vi "Pick&Place_ladder_shih_v3.vi"() -> ()   [LabVIEW 2016]
uses:
  Classes/Controllers/I-O/Copy of NI-DAQ Folder/NI-DAQ.lvclass
  D:/INTT/V1/Classes/Controllers/I-O/Copy of I-O Folder/I-O.lvclass
  Classes/Controllers/Dispenser/Copy of Ultimus V2 Folder/Ultimus V2.lvclass
  <vilib>/Analysis/coordinate.llb/2D Cartesian Coordinate Rotation (Scalar).vi
  <vilib>/Utility/file.llb/Read Delimited Spreadsheet (DBL).vi
  <vilib>/Utility/file.llb/Write Delimited Spreadsheet (DBL).vi
  Classes/Controllers/Motion/Copy of Motion Folder/Motion.lvclass
  Classes/Controllers/Camera/Copy of Controller Folder/Controller.lvclass
  <vilib>/Analysis/NI_AALPro.lvlib
  Classes/Controllers/I-O/Copy of I-O Folder/I-O.lvclass
panel:
  out "FROM Detail !!! Center of module on stave 2":dbl[](array[numeric])
  out "FROM Detail !! measured stave size":dbl[](array[numeric])
  in  "Align Stave in detail":bool
  in  "check height?":bool
  in  "Uttimus presssure":i64=10
  out "Status":bool
  out "measured HDI top-left position":dbl[][](array[numeric])
  in  "HDI vacuum channel":i32=18
  in  "vacuum":bool=TRUE
  in  "HDI vacuum":bool
  out "measured stave size":dbl[](array[numeric])
  out "Stave mark":dbl[][](array[numeric])
  out "Center of module on stave":dbl[](array[numeric])
  out "Center of HDI from alignment mark":dbl[](array[numeric])
  out "Measured HDI size":dbl[][](array[numeric])
  out "module position on stave":dbl[][](array[numeric])
  in  "Default Stave dimension":dbl[](array[numeric])=[34.0, 472.0, -0.335295, -0.000320234]
  in  "Default Stave upper left mark":dbl[](array[numeric])=[584.376, 675.576, 70.9882, 0.000840064]
  out "Needle parking position":dbl[](array[numeric])
  in  "Uppler / Lower Stave":bool=TRUE
  out "Gantry current position":dbl[](array[numeric])
  in  "READ Position":bool
  in  "Needle Height Compenstation\n(glue gap)":dbl=0.33
  in  "Needle Alignment":bool
  in  "Parking position":dbl[](array[numeric])=[625.0, 625.0, 0.0, 0.01]
  in  "GOTO":bool
  in  "Default Pickup Tool Position":dbl[][](array[numeric])=[[152.226, 682.729, 36.8129, -0.0151898], [700.0, 800.0, 20.0, 0.01]]
  in  "Number of module \nto be assembled":i32=1
  in  "Default HDI alignment \nmark position":dbl[](array[numeric])=[448.322, 976.582, 74.9872, 0.000191129]
  in  "Default HDI size":dbl[](array[numeric])=[24.2437, 231.446, -0.099339, 0.000191129]
  out "# of tasks excuted":i32
  out "module on tray position":dbl[][](array[numeric])
  out "PickupTool \nCenterPosition":dbl[](array[numeric])
  in  "Inititalize":bool
  in  "Pick and place":bool
  in  "Deposit Glue":bool
  in  "Measure Pickup Tools":bool
  in  "Align Stave":bool
  out "default module position on stave":dbl[][](array[numeric])
  in  "Stop":bool
  in  "Measure HDI":bool
  # "Ladder Assembly"
  # "Lower\nmodule"
  # "Upper\nmodule"
  # "Sensor 0.32 -> 200 micron glue thickness\nChips 0.37-> 140 micron glue thickness"
  # "ACTIONS"
  # "Stave infomation"
  # "Module infomation"
  # "Pick and Place"
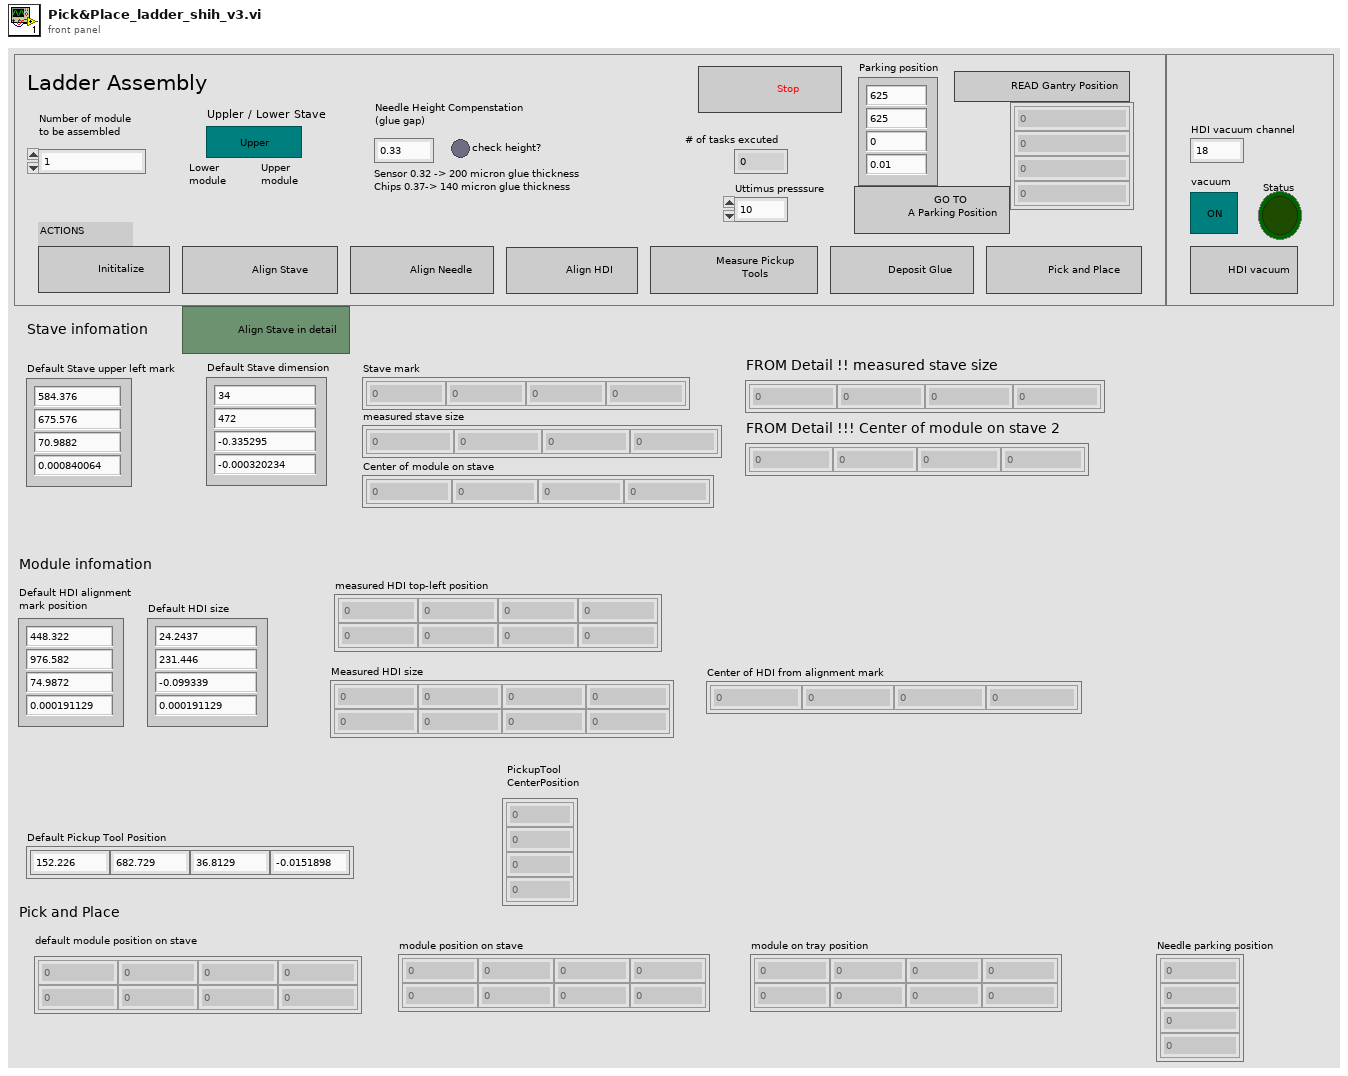
[diagram p1: front panel]
types:
  T1 = typedef "Controller.lvclass/Controllers.ctl" = cluster{"Copy of Motion.lvclass":refnum<class "Motion.lvclass">, "Copy of I-O.lvclass":refnum<class "I-O.lvclass">, "Copy of Dispenser.lvclass":refnum<class "Dispenser.lvclass">}
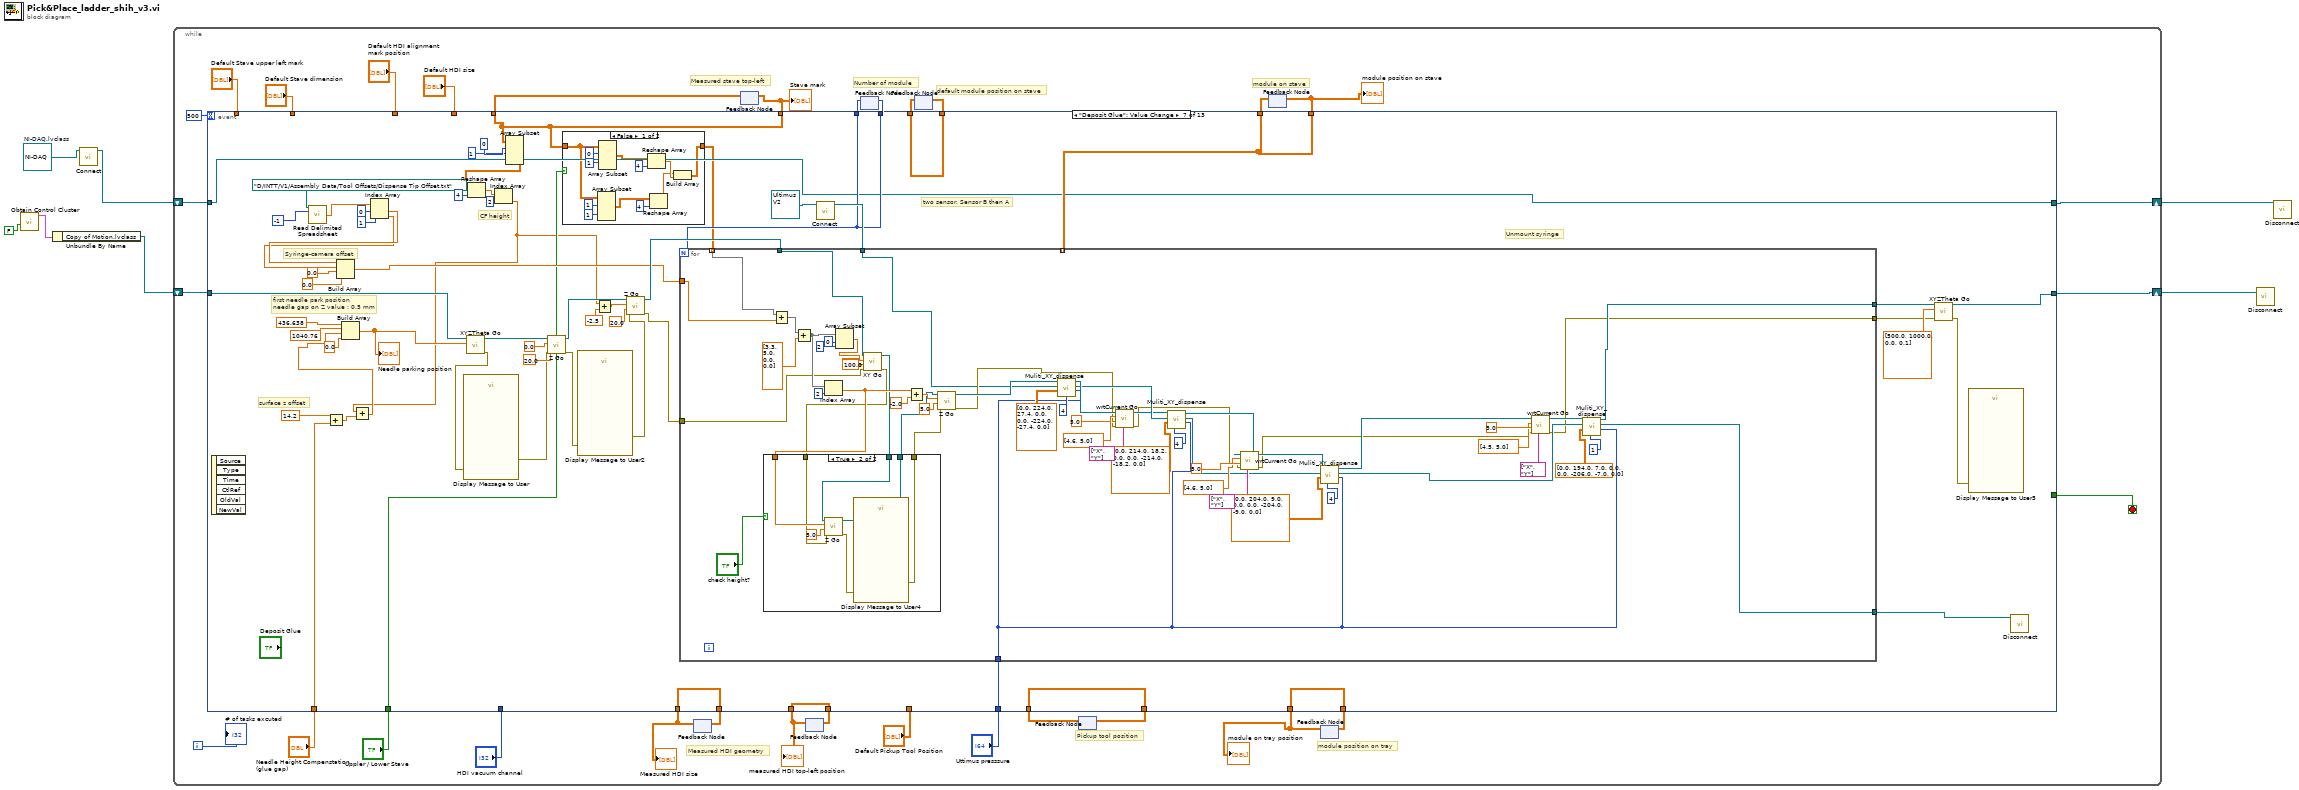
[diagram p0: block diagram]
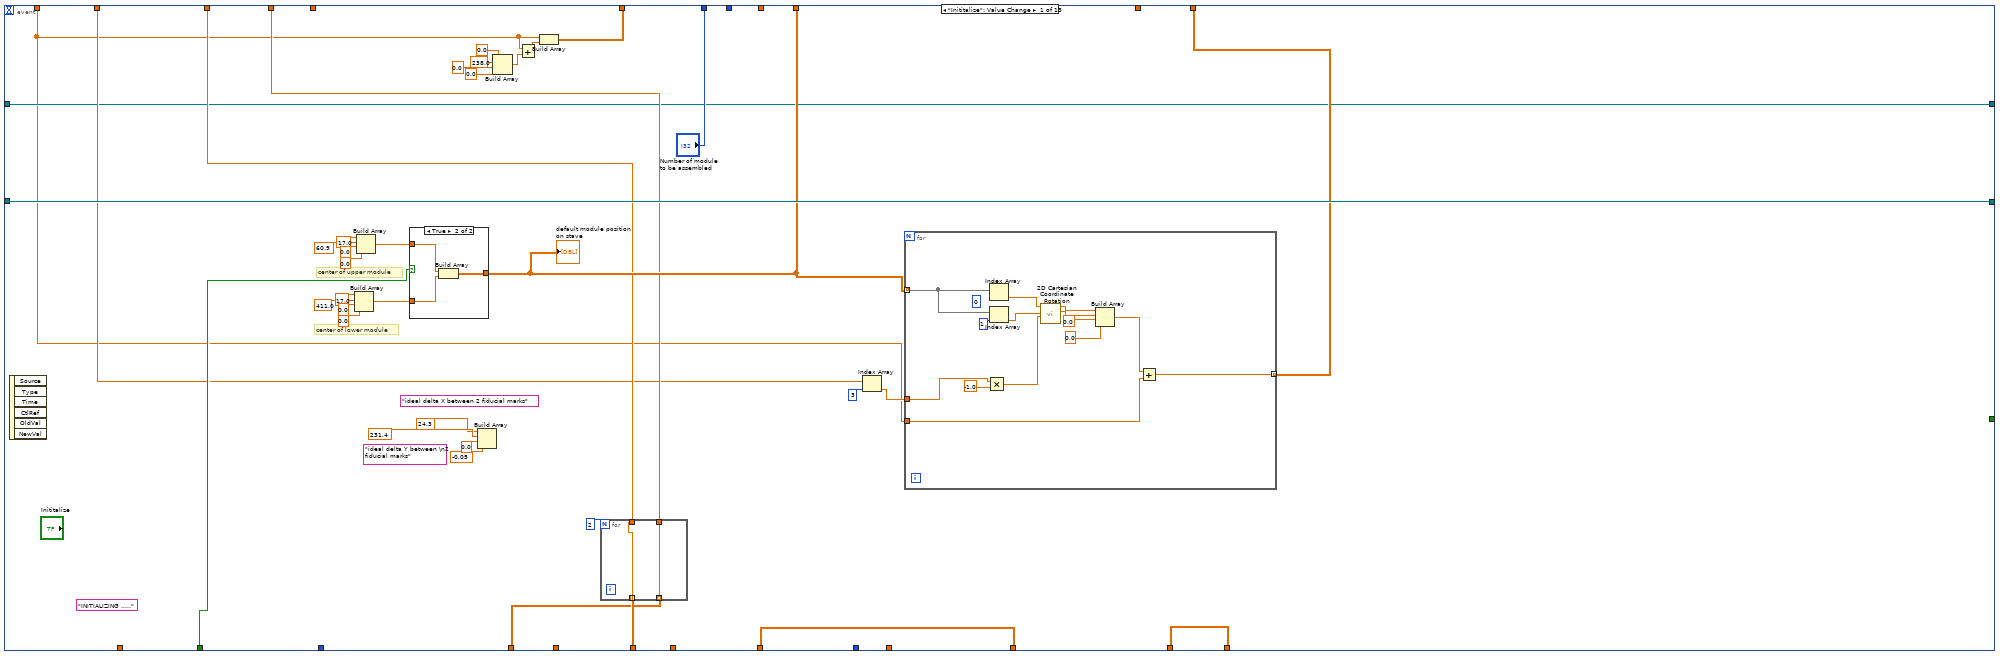
[diagram p2: hidden frame]
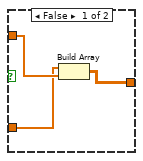
[diagram p3: hidden frame]
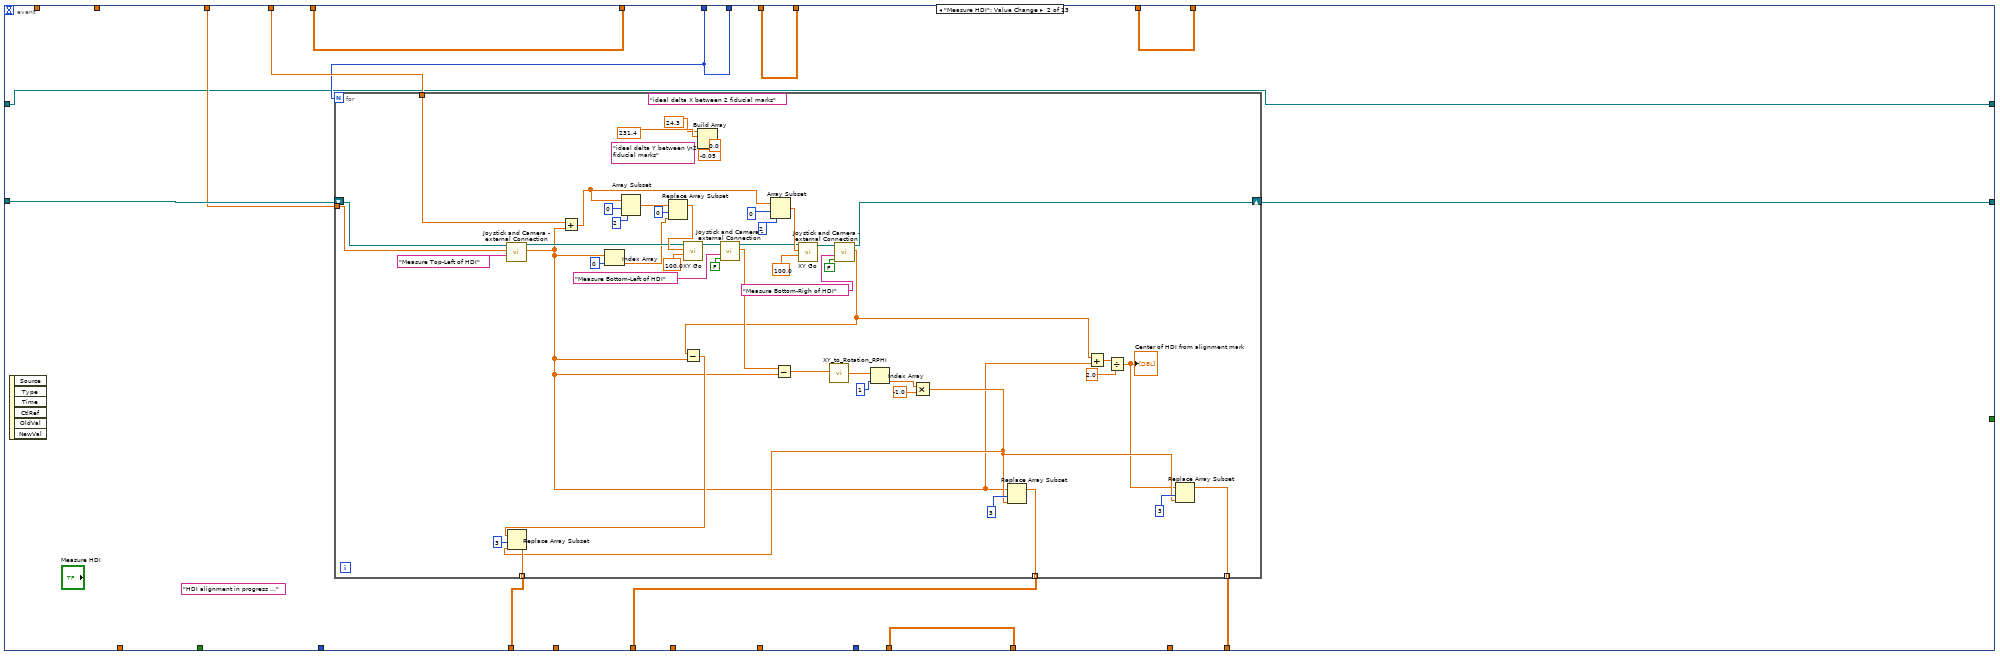
[diagram p4: hidden frame]
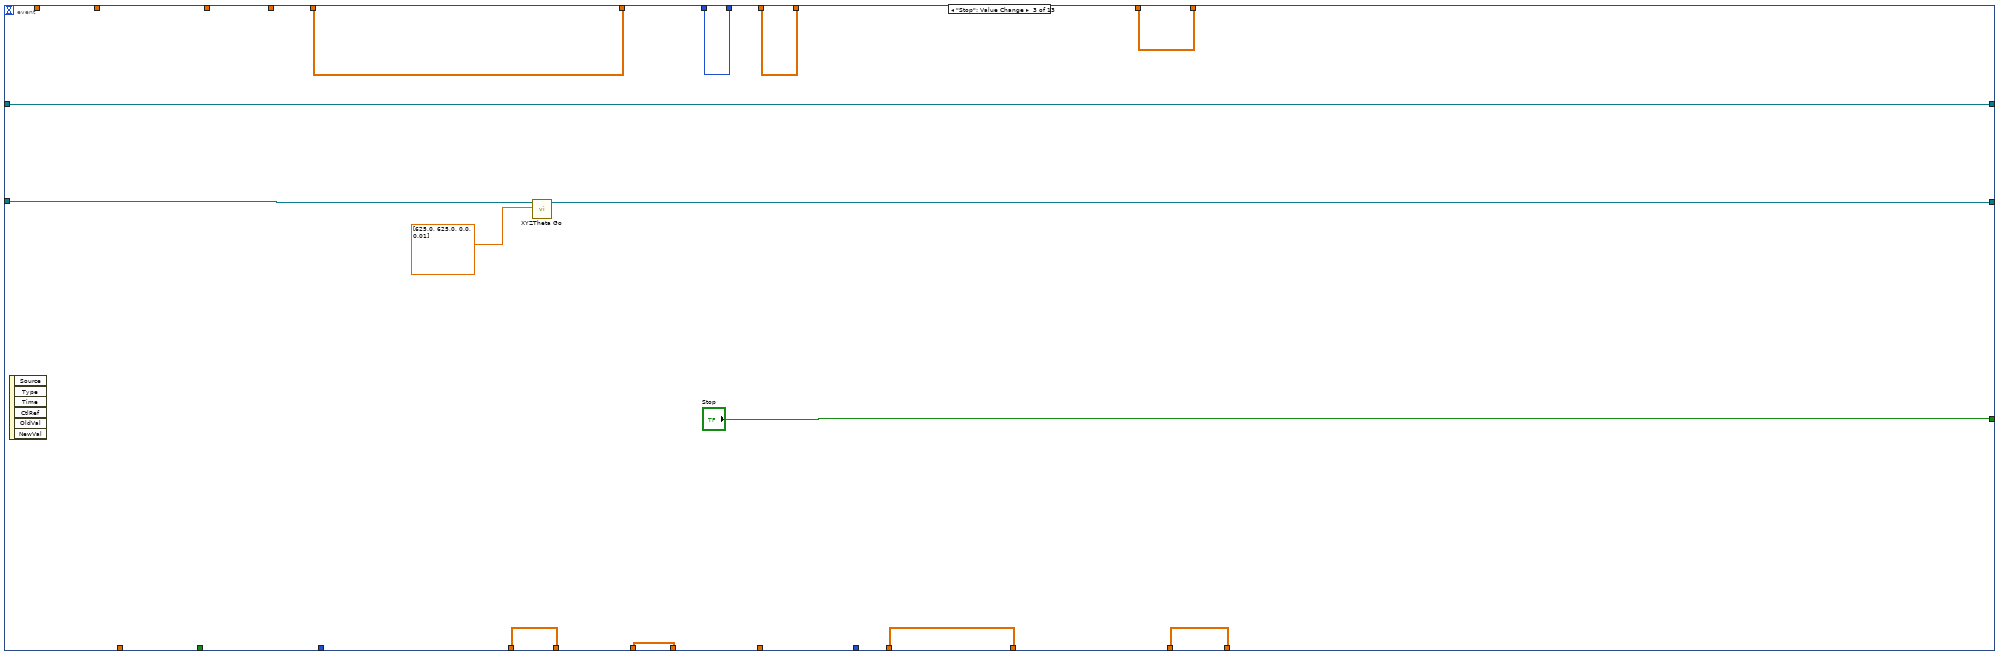
[diagram p5: hidden frame]
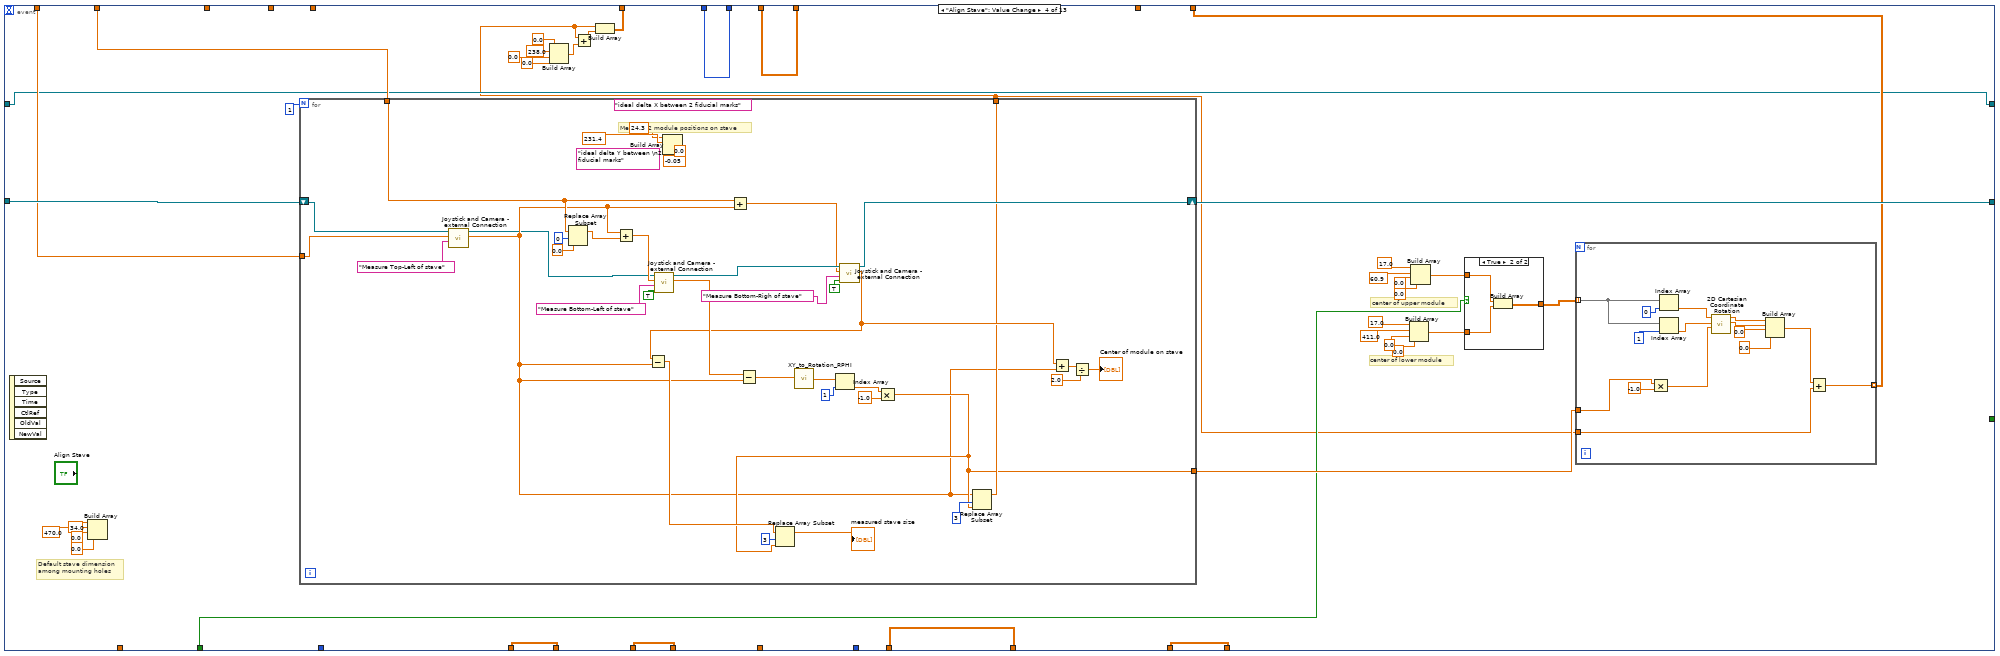
[diagram p6: hidden frame]
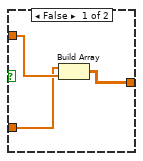
[diagram p7: hidden frame]
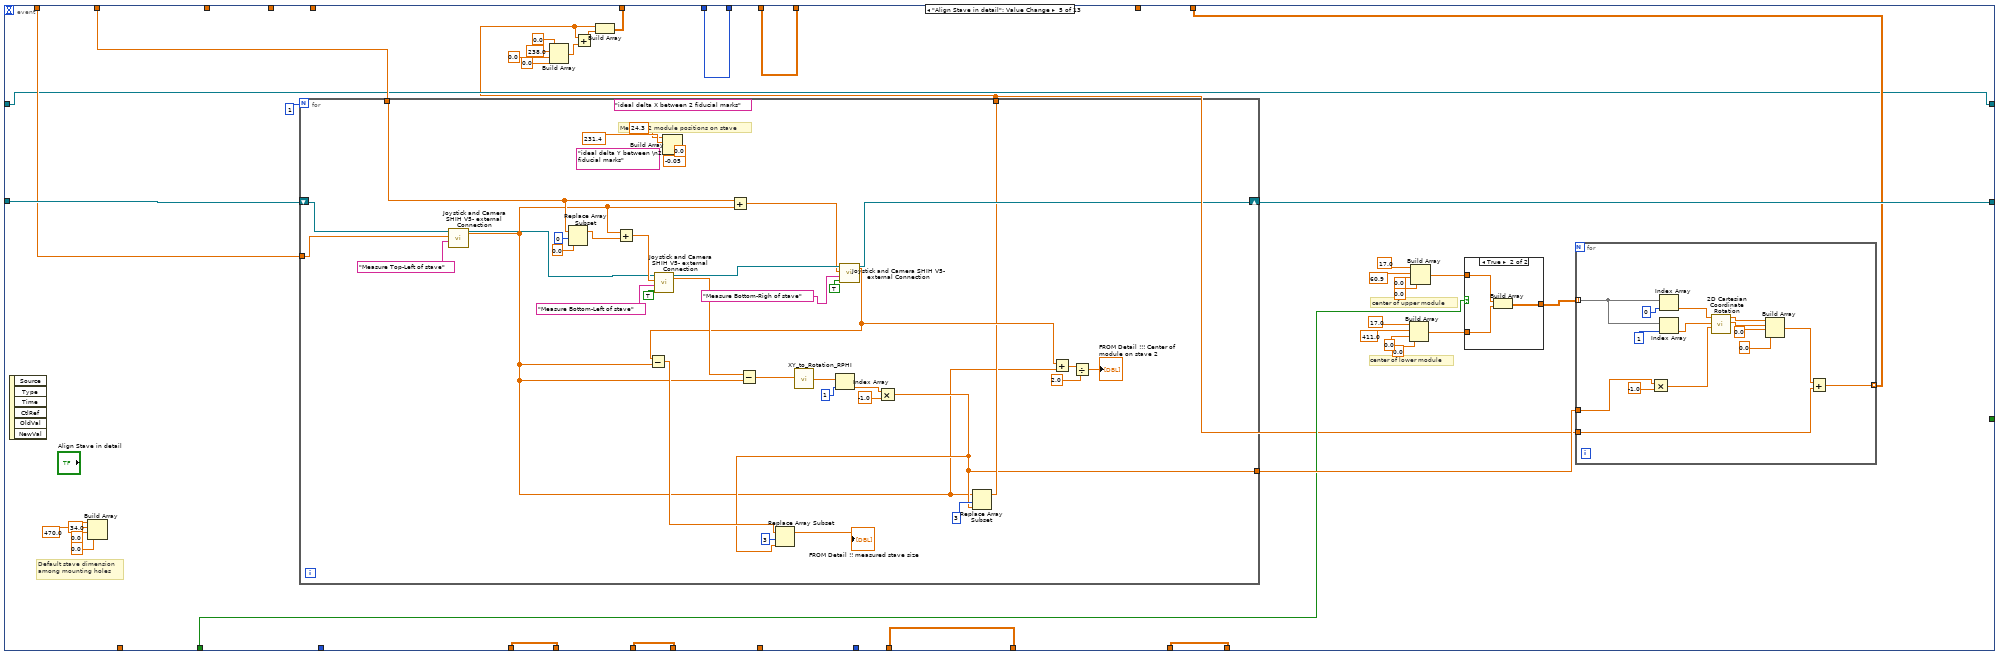
[diagram p8: hidden frame]
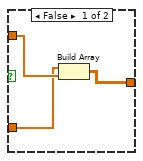
[diagram p9: hidden frame]
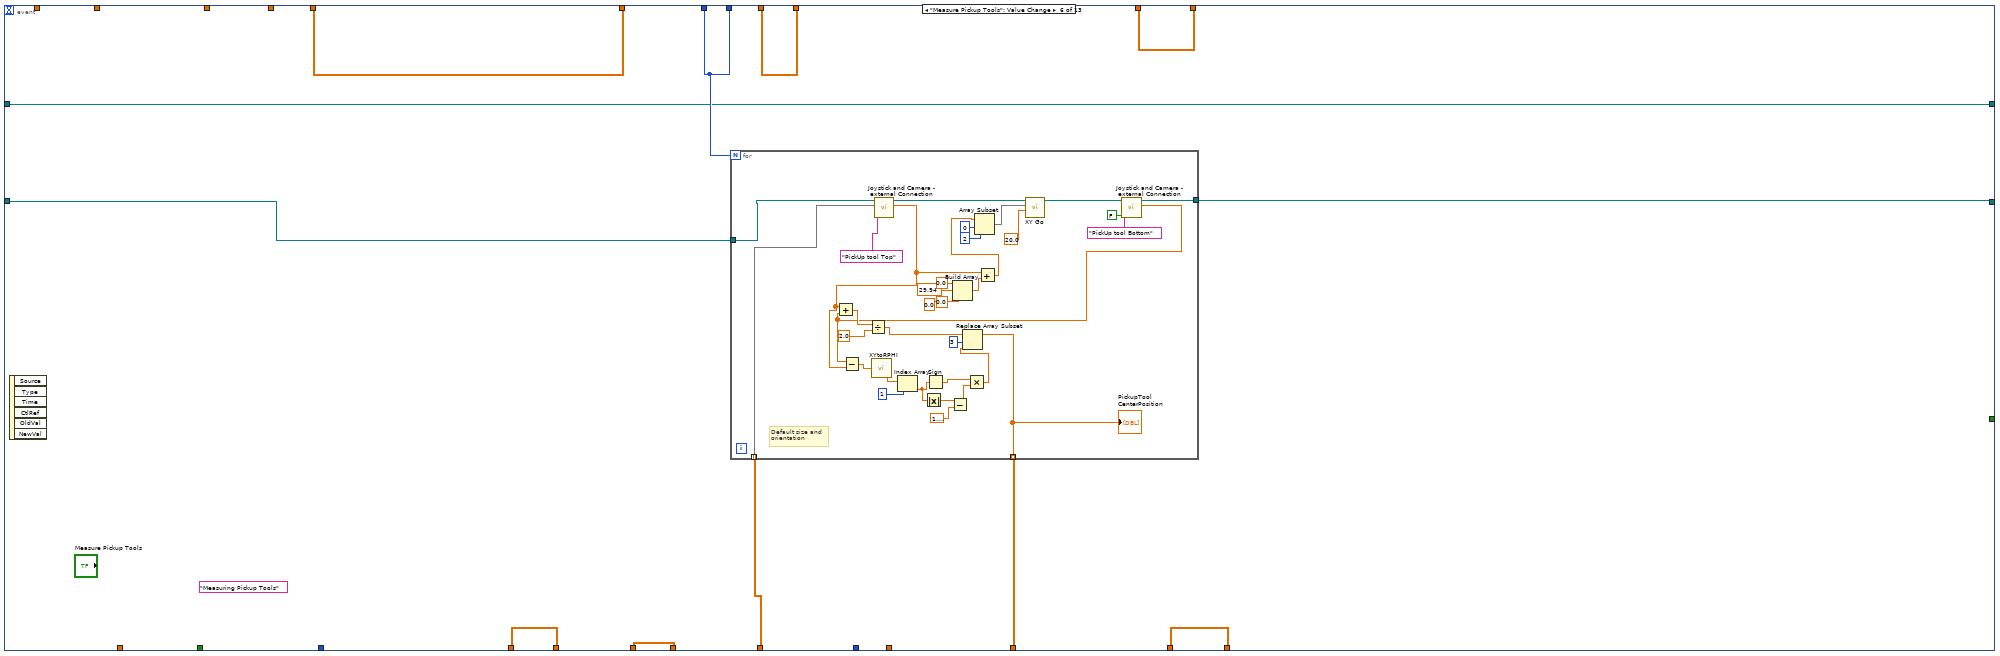
[diagram p10: hidden frame]
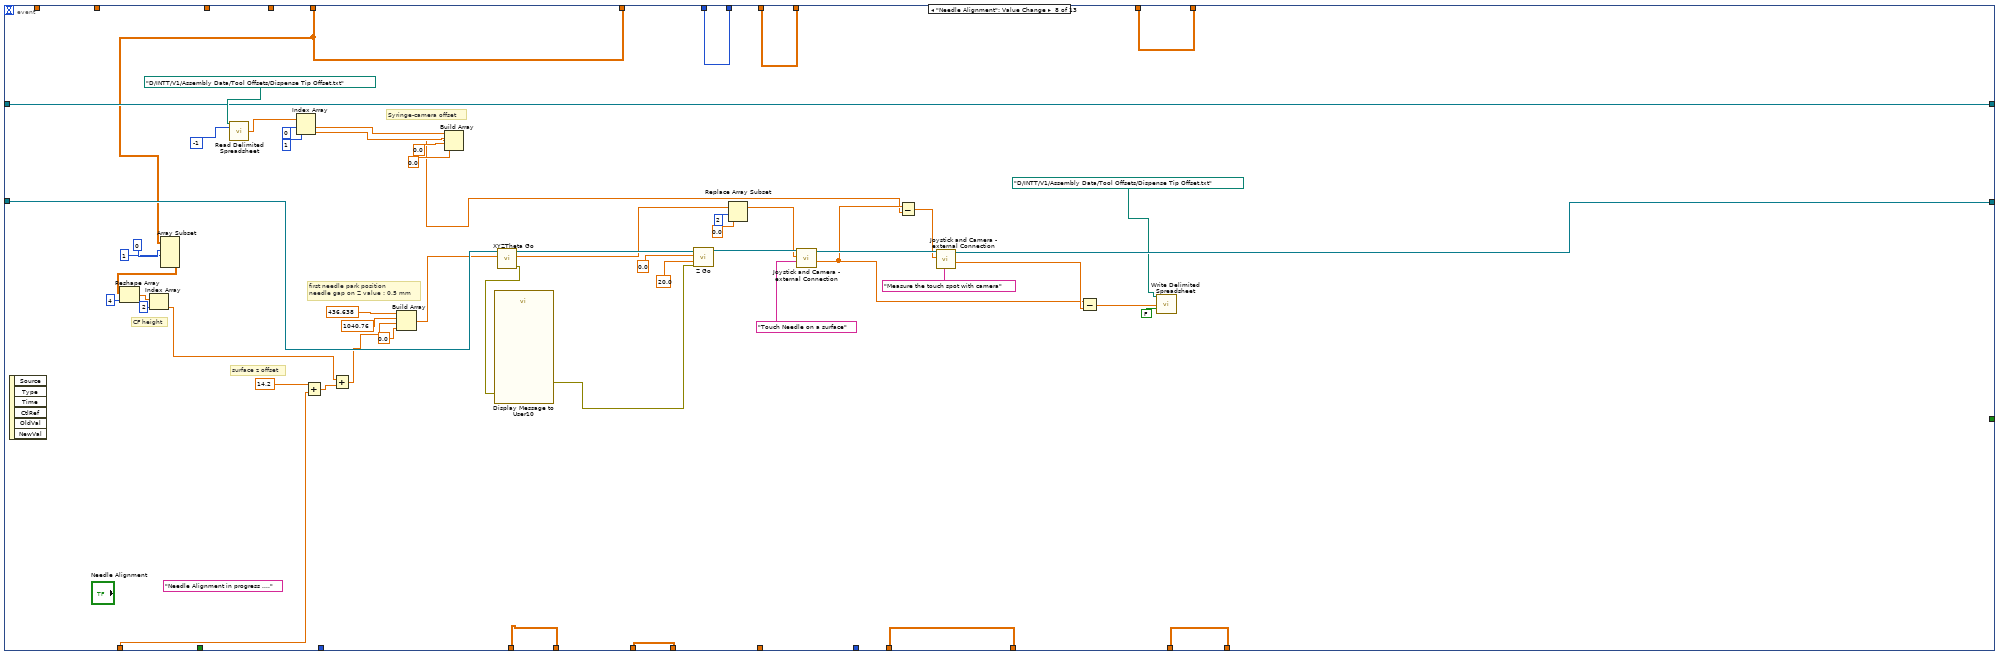
[diagram p13: hidden frame]
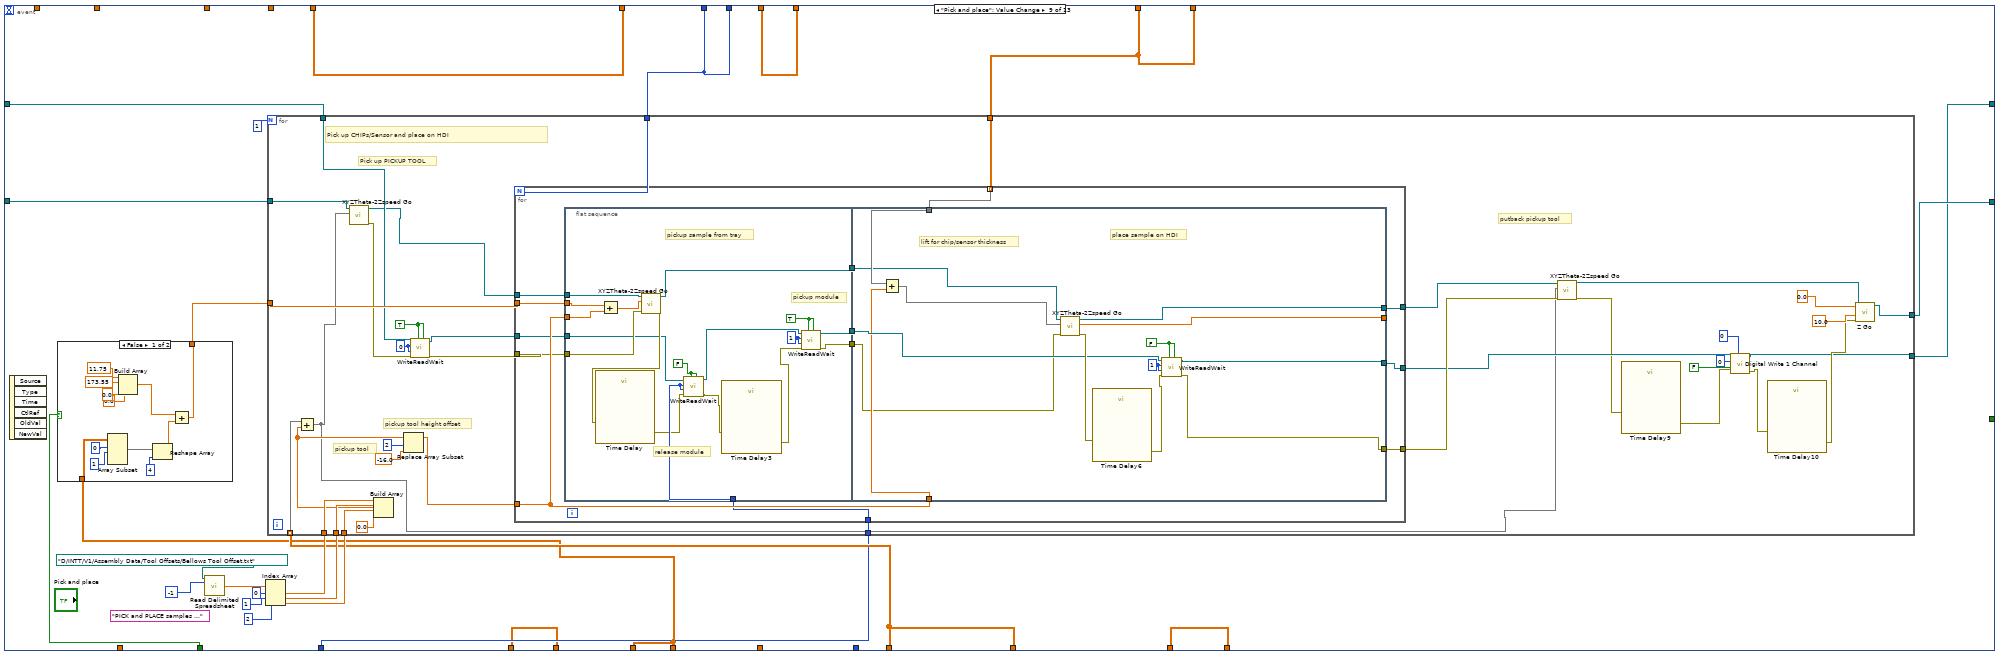
[diagram p14: hidden frame]
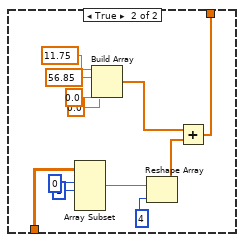
[diagram p15: hidden frame]
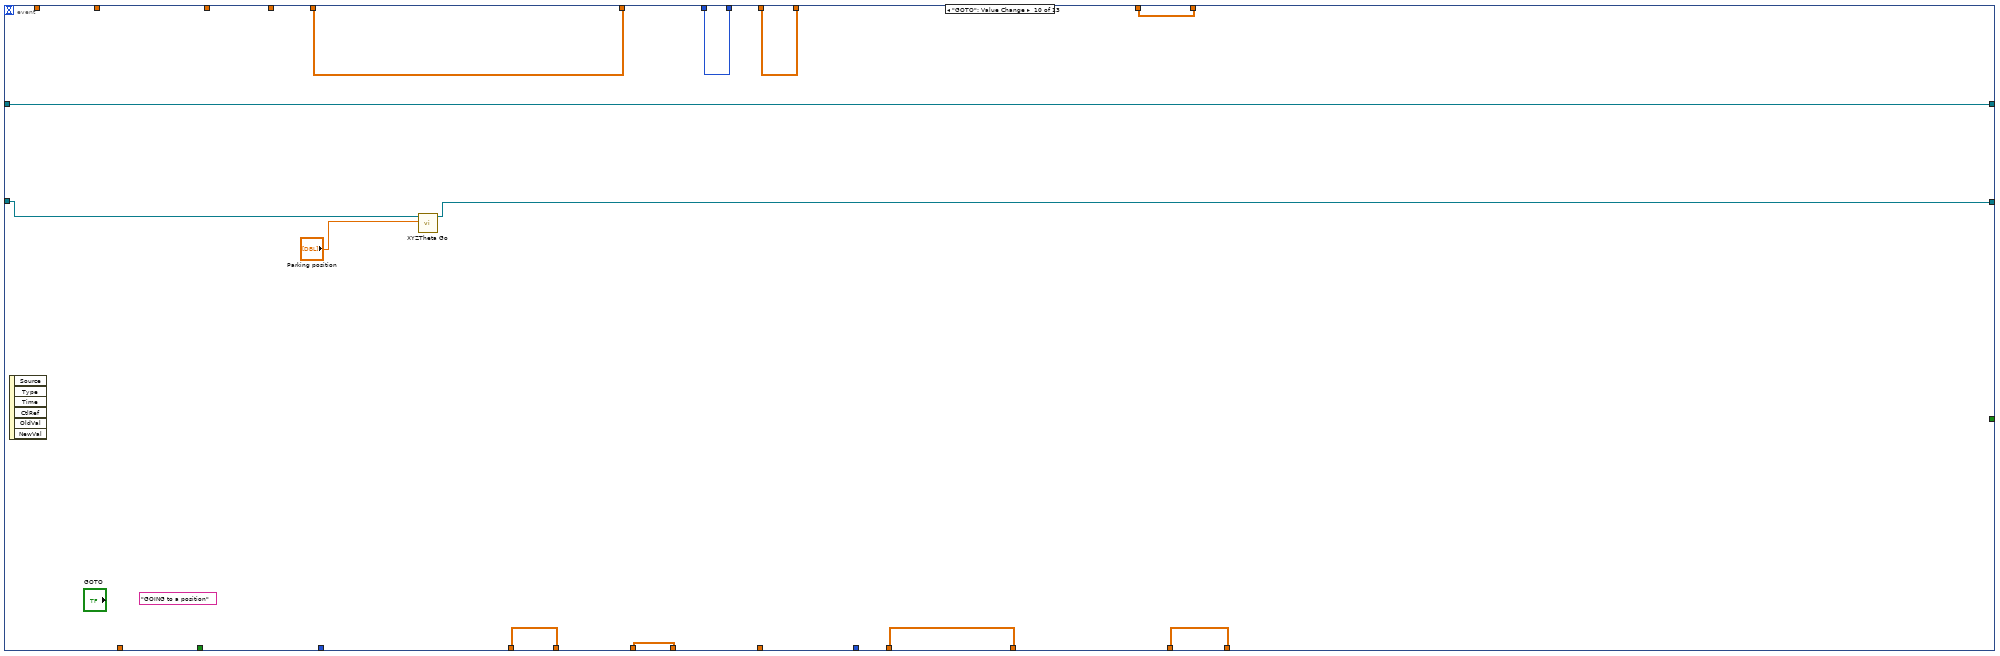
[diagram p16: hidden frame]
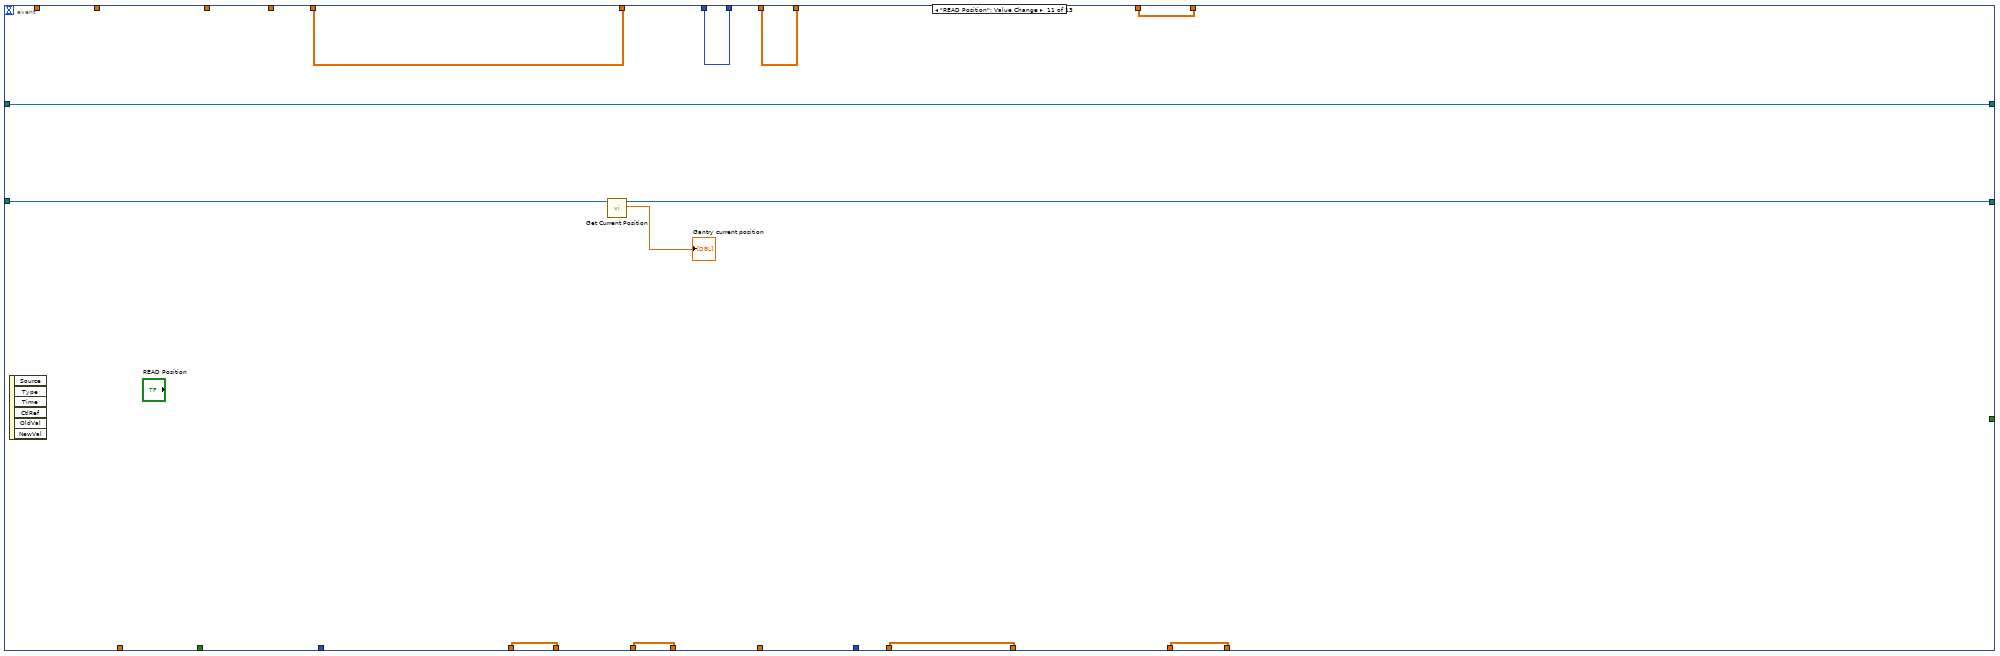
[diagram p17: hidden frame]
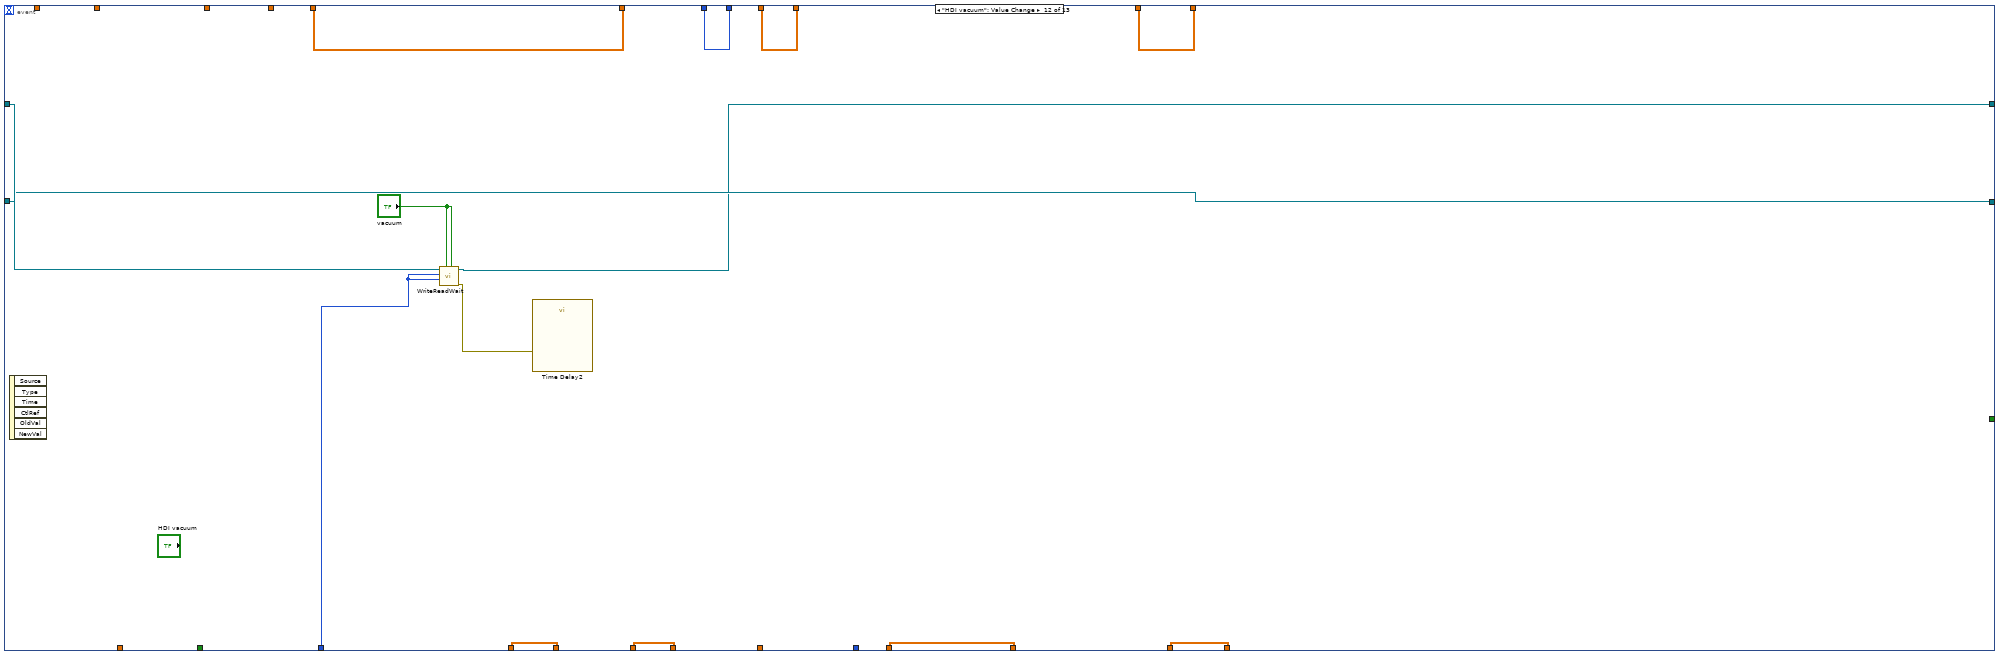
[diagram p18: hidden frame]
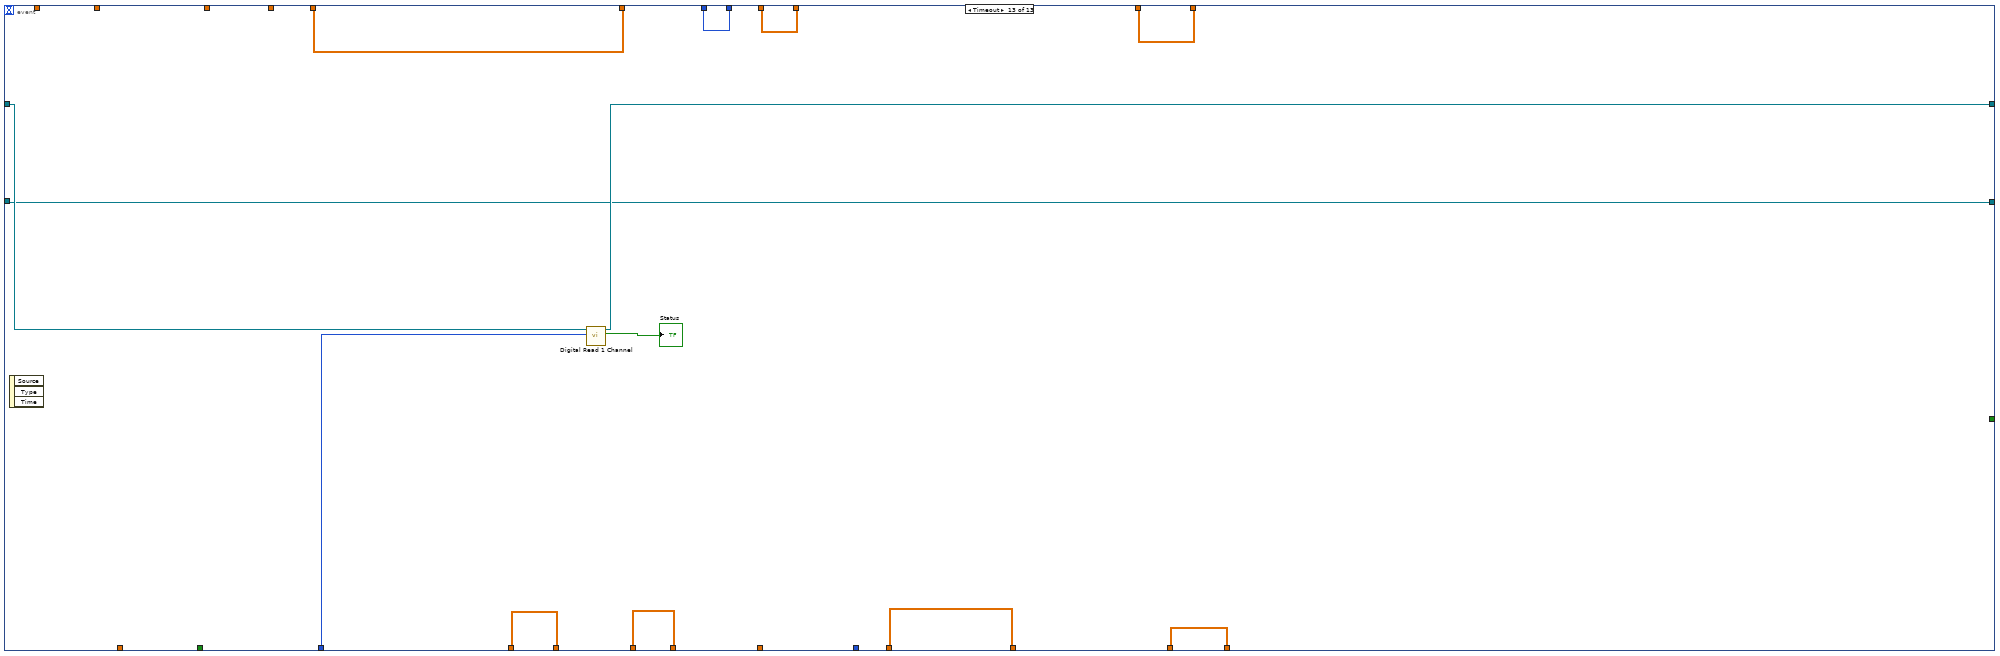
[diagram p19: hidden frame]
diagram:
  w3 = refnum<class "NI-DAQ.lvclass"> refnum  # NI-DAQ.lvclass
  n1 = call "Obtain Control Cluster.vi"("I/O"=FALSE) -> ("Control Out"=w7:T1)  [unwired: 10 in]
  n2 = Unbundle By Name(w7) -> ("Copy of Motion.lvclass"=w5:refnum<class "Motion.lvclass">)
  n3 = call-dynamic "Connect.vi"("NI-DAQ in"=w3) -> ("NI-DAQ out"=w2:refnum<class "NI-DAQ.lvclass">)  [unwired: 9 in, 1 out]
  n4 = while {
    shift-right: [w32] -> w4
    shift-left: w5 -> [w39]
    shift-right: [w11] -> w1
    shift-left: w2 -> [w15]
    i -> [w31]
    stop <- w38 stop-if-true
    # "default module position on stave"
    # "Pickup tool position"
    # "Number of module"
    # "Measured HDI geometry"
    # "module position on tray"
    # "Measured stave top-left"
    # "module on stave"
    n5 = feedback #1() -> (w36:dbl[][])  [unwired: 1 in]
    n6 = feedback #2() -> (w37:dbl[][])  [unwired: 1 in]
    n7 = feedback #3() -> (w12:dbl[][])  [unwired: 1 in]
    n8 = feedback #4() -> (w30:i32)  [unwired: 1 in]
    n9 = feedback #5() -> (w25:dbl[][])  [unwired: 1 in]
    n10 = feedback #6() -> (w33:dbl[][])  [unwired: 1 in]
    n11 = feedback #7() -> (w19:dbl[][])  [unwired: 1 in]
    n12 = feedback #8() -> (w23:dbl[][])  [unwired: 1 in]
    "module on tray position" <- w23
    n13 = event shown="[6] \"Deposit Glue\": Value Change" {
      selector: _ -> [_ _ _ _ _ _ _ _ _ _ _ _ _]
      dyn-events: _ -> [_ _ _ _ _ _ _ _ _ _ _ _ _]
      timeout: 500 -> [_ _ _ _ _ _ _ _ _ _ _ _ _]
      tunnel: w39 -> [w73 w112 w174 w204 w300 w378 w451 w585 w629 w741 w759 w761 w782]
      tunnel: [_ _ "Stop" _ _ _ _ _ _ _ _ _ _] -> w38
      tunnel: [w40 w106 w169 w175 w271 w373 w413 w551 w607 w747 w755 w769 w781] -> w16
      tunnel: w37 -> [_ w106 w169 _ _ w373 w413 w551 w607 w747 w755 w769 w781]
      tunnel: [w50 w104 w168 w200 w296 w372 w437 w588 w610 w744 w754 w763 w779] -> w17
      tunnel: w36 -> [_ _ w168 w200 w296 w372 w437 w588 w610 w744 w754 w763 w779]
      tunnel: w30 -> [_ w102 w171 w205 w301 w369 w440 w590 w614 w746 w756 w767 w774]
      tunnel: [w55 w103 w166 w207 w303 w371 w439 w586 w617 w742 w752 w765 w776] -> w35
      tunnel: w23 -> [w55 _ w166 w207 w303 w371 w439 w586 w617 w742 w752 w765 w776]
      tunnel: [w71 w107 w167 w212 w308 w377 w438 w587 w618 w743 w753 w764 w777] -> w34
      tunnel: w33 -> [_ w107 w167 w212 w308 _ w438 w587 w618 w743 w753 w764 w777]
      tunnel: [w73 w111 w172 w201 w297 w376 w441 w577 w619 w739 w758 w761 w782] -> w32
      tunnel: ["Number of module \nto be assembled" w102 w171 w205 w301 w369 w440 w590 w614 w746 w756 w767 w774] -> w29
      tunnel: "Default HDI alignment \nmark position" -> [w53 w110 _ _ _ _ _ _ _ _ _ _ _]
      tunnel: "Default HDI size" -> [w52 w109 _ _ _ _ _ _ _ _ _ _ _]
      tunnel: [w60 w108 w170 w206 w302 w374 w436 w589 w616 w745 w757 w768 w780] -> w26
      tunnel: w25 -> [_ w108 w170 w206 w302 w374 w436 w589 w616 w745 w757 w768 w780]
      tunnel: "Default Pickup Tool Position" -> [w71 _ _ _ _ w375 _ _ _ _ _ _ _]
      tunnel: "Uppler / Lower Stave" -> [w56 _ _ w185 w281 _ w421 _ w605 _ _ _ _]
      tunnel: "Default Stave upper left mark" -> [w41 _ _ w203 w299 _ _ _ _ _ _ _ _]
      tunnel: "Default Stave dimension" -> [w49 _ _ w202 w298 _ _ _ _ _ _ _ _]
      tunnel: [w57 w105 w164 w184 w280 w370 w435 w568 w606 w737 w749 w766 w775] -> w18
      tunnel: w19 -> [_ w105 w164 _ _ w370 w435 w568 w606 w737 w749 w766 w775]
      tunnel: w15 -> [w48 w100 w162 w183 w279 w367 w430 w566 w613 w736 w748 w773 w785]
      tunnel: [w48 w100 w162 w183 w279 w367 w430 w566 w612 w736 w748 w760 w783] -> w11
      tunnel: "HDI vacuum channel" -> [_ _ _ _ _ _ _ _ w611 _ _ w770 w784]
      tunnel: [w51 w101 w163 w199 w295 w368 w431 w567 w609 w738 w750 w762 w778] -> w13
      tunnel: w12 -> [_ _ w163 w199 w295 w368 w431 w567 w609 w738 w750 w762 w778]
      tunnel: "Needle Height Compenstation\n(glue gap)" -> [_ _ _ _ _ _ w423 w559 _ _ _ _ _]
      tunnel: "Uttimus presssure" -> [_ _ _ _ _ _ w422 _ _ _ _ _ _]
      event "Inititalize": Value Change {
        (unwired) "INITIALIZING ....." ("String")
        (unwired) "ideal delta Y between \n2 fiducial marks"
        (unwired) "ideal delta X between 2 fiducial marks"
        # "center of lower module"
        # "center of upper module"
        n14 = event-data() -> ()  [unwired: 1 in, 6 out]
        n15 = Build Array(17.0 ("element"), 411.0 ("element"), 0.0 ("element"), 0.0 ("element")) -> (w61:dbl[])
        n16 = Build Array(17.0 ("element"), 60.9 ("element"), 0.0 ("element"), 0.0 ("element")) -> (w62:dbl[])
        n17 = case shown="True" w56 {
          tunnel: w62 -> [w82 w85]
          tunnel: w61 -> [w81 w84]
          tunnel: [w80 w83] -> w60
          frame False {
            n18 = Build Array(w81, w82) -> (w80:dbl[][])
          }
          frame True {
            n19 = Build Array(w85, w84) -> (w83:dbl[][])
          }
        }
        "default module position on stave" <- w60
        n20 = Build Array(24.3 ("y"), 231.4 ("y"), 0.0 ("element"), -0.05 ("element")) -> ()  [unwired: 1 out]
        n21 = Build Array(0.0 ("element"), 238.0 ("element"), 0.0 ("element"), 0.0 ("element")) -> (w43:dbl[])
        n22 = Add(x=w41, y=w43) -> (x+y=w42:dbl[])
        n23 = Build Array(w41, w42) -> (w40:dbl[][])
        n24 = for {
          N: 2 -> [_]
          tunnel: w53 -> [w79]
          tunnel: [w79] -> w51 mode=indexing
          tunnel: w52 -> [w78]
          tunnel: [w78] -> w50 mode=indexing
        }
        n25 = Index Array(array=w49, index=3) -> (element=w58:dbl)
        n26 = for {
          tunnel: w60 -> [w93] mode=indexing
          tunnel: w58 -> [w87]
          tunnel: w41 -> [w92]
          tunnel: [w90] -> w57 mode=indexing
          (unwired) 0 ("index")
          n27 = Multiply(x=w87, y=-1.0) -> (x*y=w88:dbl)
          n28 = Index Array(array=w93) -> (element=w96:dbl)  [unwired: 1 in]
          n29 = Index Array(array=w93, index=1) -> (element=w95:dbl)
          n30 = call-poly <vilib>:"2D Cartesian Coordinate Rotation.vi"("theta"=w88, "y"=w95, "x"=w96) -> ("y out"=w98:dbl, "x out"=w97:dbl)  [unwired: 6 in, 1 out]
          n31 = Build Array(w97, w98, 0.0 ("element"), 0.0 ("element")) -> (w91:dbl[])
          n32 = Add(x=w91, y=w92) -> (x+y=w90:dbl[])
        }
      }
      event "Measure HDI": Value Change {
        (unwired) "HDI alignment in progress ..." ("String")
        n33 = event-data() -> ()  [unwired: 1 in, 6 out]
        n34 = for {
          N: w102 -> [_]
          tunnel: w109 -> [w124]
          shift-right: [w121] -> w111
          shift-left: w112 -> [w122]
          tunnel: w110 -> [w123]
          tunnel: [w158] -> w101 mode=indexing
          tunnel: [w157] -> w104 mode=indexing
          tunnel: [w114] -> w103 mode=indexing
          (unwired) "ideal delta Y between \n2 fiducial marks"
          (unwired) "ideal delta X between 2 fiducial marks"
          n35 = call "Joystick and Camera - external Connection.vi"("Motion in"=w122, "XYZTheta"=w123, "Measurement Point"="Measure Top-Left of HDI") -> ("Motion out"=w137:refnum<class "Motion.lvclass">, "Sum"=w113:dbl[])  [unwired: 4 in, 2 out]
          n36 = Add(x=w124, y=w113) -> (x+y=w141:dbl[])
          n37 = Index Array(array=w113, index=0) -> (element=w128:dbl)
          n38 = Array Subset(array=w141, index=0, length=2) -> (w140:dbl[])
          n39 = Replace Array Subset(array=w140, new element=w128, index=0) -> (w138:dbl[])
          n40 = call-dynamic "XY Go.vi"("Speed"=100.0, "XY"=w138, "Motion in"=w137) -> ("Motion out"=w145:refnum<class "Motion.lvclass">)  [unwired: 7 in, 1 out]
          n41 = Build Array(24.3 ("y"), 231.4 ("y"), 0.0 ("element"), -0.05 ("element")) -> ()  [unwired: 1 out]
          n42 = call "Joystick and Camera - external Connection.vi"("Motion in"=w145, "Measurement Point"="Measure Bottom-Left of HDI", "Inital GO"=FALSE) -> ("Motion out"=w136:refnum<class "Motion.lvclass">, "Sum"=w127:dbl[])  [unwired: 4 in, 2 out]
          n43 = Array Subset(array=w141, index=0, length=2) -> (w151:dbl[])
          n44 = Subtract(x=w127, y=w113) -> (x-y=w135:dbl[])
          n45 = call-dynamic "XY Go.vi"("Speed"=100.0, "XY"=w151, "Motion in"=w136) -> ("Motion out"=w155:refnum<class "Motion.lvclass">)  [unwired: 7 in, 1 out]
          n46 = call "XY_to_Rotation_RPHI.vi"("X-Y"=w135) -> ("r-phi"=w131:dbl[])
          n47 = call "Joystick and Camera - external Connection.vi"("Motion in"=w155, "Measurement Point"="Measure Bottom-Righ of HDI", "Inital GO"=FALSE) -> ("Motion out"=w121:refnum<class "Motion.lvclass">, "Sum"=w118:dbl[])  [unwired: 4 in, 2 out]
          n48 = Subtract(x=w118, y=w113) -> (x-y=w119:dbl[])
          n49 = Index Array(array=w131, index=1) -> (element=w125:dbl)
          n50 = Multiply(x=w125, y=-1.0) -> (x*y=w116:dbl)
          n51 = Replace Array Subset(array=w119, new element=w116, index=3) -> (w157:dbl[])
          n52 = Replace Array Subset(array=w113, new element=w116, index=3) -> (w158:dbl[])
          n53 = Add(x=w118, y=w113) -> (x+y=w160:dbl[])
          n54 = Divide(x=w160, y=2.0) -> (x/y=w115:dbl[])
          "Center of HDI from alignment mark" <- w115
          n55 = Replace Array Subset(array=w115, new element=w116, index=3) -> (w114:dbl[])
        }
      }
      event "Stop": Value Change {
        n56 = event-data() -> ()  [unwired: 1 in, 6 out]
        n57 = call "XYZTheta Go.vi"("XYZTheta In"=dbl[] [625.0, 625.0, 0.0, 0.01], "Motion in"=w174) -> ("Motion out"=w172:refnum<class "Motion.lvclass">)  [unwired: 7 in, 2 out]
      }
      event "Align Stave": Value Change {
        # "center of lower module"
        # "center of upper module"
        # "Default stave dimension\namong mounting holes"
        # "Measure 2 module positions on stave"
        n58 = event-data() -> ()  [unwired: 1 in, 6 out]
        n59 = Build Array(34.0 ("element"), 470.0 ("element"), 0.0 ("element"), 0.0 ("element")) -> ()  [unwired: 1 out]
        n60 = for {
          N: 1 -> [_]
          tunnel: w202 -> [w240]
          shift-right: [w250] -> w201
          shift-left: w204 -> [w251]
          tunnel: w203 -> [w252]
          tunnel: [w245] -> w177
          tunnel: [w243] -> w187
          (unwired) "ideal delta Y between \n2 fiducial marks"
          (unwired) "ideal delta X between 2 fiducial marks"
          n61 = call "Joystick and Camera - external Connection.vi"("Motion in"=w251, "XYZTheta"=w252, "Measurement Point"="Measure Top-Left of stave") -> ("Motion out"=w234:refnum<class "Motion.lvclass">, "Sum"=w236:dbl[])  [unwired: 4 in, 2 out]
          n62 = Replace Array Subset(array=w240, new element=0.0 ("new element/subarray"), index=0) -> (w237:dbl[])
          n63 = Add(x=w236, y=w237) -> (x+y=w235:dbl[])
          n64 = call "Joystick and Camera - external Connection.vi"("Motion in"=w234, "XYZTheta"=w235, "Measurement Point"="Measure Bottom-Left of stave", "Inital GO"=TRUE) -> ("Motion out"=w242:refnum<class "Motion.lvclass">, "Sum"=w255:dbl[])  [unwired: 3 in, 2 out]
          n65 = Build Array(24.3 ("y"), 231.4 ("y"), 0.0 ("element"), -0.05 ("element")) -> ()  [unwired: 1 out]
          n66 = Add(x=w240, y=w236) -> (x+y=w241:dbl[])
          n67 = Subtract(x=w255, y=w236) -> (x-y=w261:dbl[])
          n68 = call "XY_to_Rotation_RPHI.vi"("X-Y"=w261) -> ("r-phi"=w257:dbl[])
          n69 = Index Array(array=w257, index=1) -> (element=w253:dbl)
          n70 = call "Joystick and Camera - external Connection.vi"("Motion in"=w242, "XYZTheta"=w241, "Measurement Point"="Measure Bottom-Righ of stave", "Inital GO"=TRUE) -> ("Motion out"=w250:refnum<class "Motion.lvclass">, "Sum"=w247:dbl[])  [unwired: 3 in, 2 out]
          n71 = Subtract(x=w247, y=w236) -> (x-y=w248:dbl[])
          n72 = Multiply(x=w253, y=-1.0) -> (x*y=w243:dbl)
          n73 = Replace Array Subset(array=w248, new element=w243, index=3) -> (→"measured stave size":dbl[])
          n74 = Replace Array Subset(array=w236, new element=w243, index=3) -> (w245:dbl[])
          n75 = Add(x=w247, y=w236) -> (x+y=w269:dbl[])
          n76 = Divide(x=w269, y=2.0) -> (x/y=→"Center of module on stave":dbl[])
        }
        n77 = Build Array(0.0 ("element"), 238.0 ("element"), 0.0 ("element"), 0.0 ("element")) -> (w178:dbl[])
        n78 = Add(x=w177, y=w178) -> (x+y=w176:dbl[])
        n79 = Build Array(w177, w176) -> (w175:dbl[][])
        n80 = Build Array(17.0 ("element"), 411.0 ("element"), 0.0 ("element"), 0.0 ("element")) -> (w189:dbl[])
        n81 = Build Array(17.0 ("element"), 60.9 ("element"), 0.0 ("element"), 0.0 ("element")) -> (w190:dbl[])
        n82 = case shown="True" w185 {
          tunnel: w190 -> [w230 w233]
          tunnel: w189 -> [w229 w232]
          tunnel: [w228 w231] -> w188
          frame False {
            n83 = Build Array(w229, w230) -> (w228:dbl[][])
          }
          frame True {
            n84 = Build Array(w233, w232) -> (w231:dbl[][])
          }
        }
        n85 = for {
          tunnel: w188 -> [w221] mode=indexing
          tunnel: w187 -> [w216]
          tunnel: w177 -> [w220]
          tunnel: [w218] -> w184 mode=indexing
          n86 = Multiply(x=w216, y=-1.0) -> (x*y=w215:dbl)
          n87 = Index Array(array=w221, index=0) -> (element=w224:dbl)
          n88 = Index Array(array=w221, index=1) -> (element=w223:dbl)
          n89 = call-poly <vilib>:"2D Cartesian Coordinate Rotation.vi"("theta"=w215, "y"=w223, "x"=w224) -> ("y out"=w226:dbl, "x out"=w225:dbl)  [unwired: 6 in, 1 out]
          n90 = Build Array(w225, w226, 0.0 ("element"), 0.0 ("element")) -> (w219:dbl[])
          n91 = Add(x=w219, y=w220) -> (x+y=w218:dbl[])
        }
      }
      event "Align Stave in detail": Value Change {
        # "center of lower module"
        # "center of upper module"
        # "Default stave dimension\namong mounting holes"
        # "Measure 2 module positions on stave"
        n92 = event-data() -> ()  [unwired: 1 in, 6 out]
        n93 = Build Array(34.0 ("element"), 470.0 ("element"), 0.0 ("element"), 0.0 ("element")) -> ()  [unwired: 1 out]
        n94 = for {
          N: 1 -> [_]
          tunnel: w298 -> [w336]
          shift-right: [w346] -> w297
          shift-left: w300 -> [w347]
          tunnel: w299 -> [w348]
          tunnel: [w341] -> w273
          tunnel: [w339] -> w283
          (unwired) "ideal delta Y between \n2 fiducial marks"
          (unwired) "ideal delta X between 2 fiducial marks"
          n95 = call "Joystick and Camera SHIH V5- external Connection.vi"("Motion in"=w347, "XYZTheta"=w348, "Measurement Point"="Measure Top-Left of stave") -> ("final out"=w332:dbl[], "Motion out"=w330:refnum<class "Motion.lvclass">)  [unwired: 5 in, 1 out]
          n96 = Replace Array Subset(array=w336, new element=0.0 ("new element/subarray"), index=0) -> (w333:dbl[])
          n97 = Add(x=w332, y=w333) -> (x+y=w331:dbl[])
          n98 = call "Joystick and Camera SHIH V5- external Connection.vi"("Motion in"=w330, "XYZTheta"=w331, "Measurement Point"="Measure Bottom-Left of stave", "Inital GO"=TRUE) -> ("final out"=w351:dbl[], "Motion out"=w338:refnum<class "Motion.lvclass">)  [unwired: 4 in, 1 out]
          n99 = Build Array(24.3 ("y"), 231.4 ("y"), 0.0 ("element"), -0.05 ("element")) -> ()  [unwired: 1 out]
          n100 = Add(x=w336, y=w332) -> (x+y=w337:dbl[])
          n101 = Subtract(x=w351, y=w332) -> (x-y=w357:dbl[])
          n102 = call "XY_to_Rotation_RPHI.vi"("X-Y"=w357) -> ("r-phi"=w353:dbl[])
          n103 = Index Array(array=w353, index=1) -> (element=w349:dbl)
          n104 = call "Joystick and Camera SHIH V5- external Connection.vi"("Motion in"=w338, "XYZTheta"=w337, "Measurement Point"="Measure Bottom-Righ of stave", "Inital GO"=TRUE) -> ("final out"=w343:dbl[], "Motion out"=w346:refnum<class "Motion.lvclass">)  [unwired: 4 in, 1 out]
          n105 = Subtract(x=w343, y=w332) -> (x-y=w344:dbl[])
          n106 = Multiply(x=w349, y=-1.0) -> (x*y=w339:dbl)
          n107 = Replace Array Subset(array=w344, new element=w339, index=3) -> (→"FROM Detail !! measured stave size":dbl[])
          n108 = Replace Array Subset(array=w332, new element=w339, index=3) -> (w341:dbl[])
          n109 = Add(x=w343, y=w332) -> (x+y=w365:dbl[])
          n110 = Divide(x=w365, y=2.0) -> (x/y=→"FROM Detail !!! Center of module on stave 2":dbl[])
        }
        n111 = Build Array(0.0 ("element"), 238.0 ("element"), 0.0 ("element"), 0.0 ("element")) -> (w274:dbl[])
        n112 = Add(x=w273, y=w274) -> (x+y=w272:dbl[])
        n113 = Build Array(w273, w272) -> (w271:dbl[][])
        n114 = Build Array(17.0 ("element"), 411.0 ("element"), 0.0 ("element"), 0.0 ("element")) -> (w285:dbl[])
        n115 = Build Array(17.0 ("element"), 60.9 ("element"), 0.0 ("element"), 0.0 ("element")) -> (w286:dbl[])
        n116 = case shown="True" w281 {
          tunnel: w286 -> [w326 w329]
          tunnel: w285 -> [w325 w328]
          tunnel: [w324 w327] -> w284
          frame False {
            n117 = Build Array(w325, w326) -> (w324:dbl[][])
          }
          frame True {
            n118 = Build Array(w329, w328) -> (w327:dbl[][])
          }
        }
        n119 = for {
          tunnel: w284 -> [w317] mode=indexing
          tunnel: w283 -> [w312]
          tunnel: w273 -> [w316]
          tunnel: [w314] -> w280 mode=indexing
          n120 = Multiply(x=w312, y=-1.0) -> (x*y=w311:dbl)
          n121 = Index Array(array=w317, index=0) -> (element=w320:dbl)
          n122 = Index Array(array=w317, index=1) -> (element=w319:dbl)
          n123 = call-poly <vilib>:"2D Cartesian Coordinate Rotation.vi"("theta"=w311, "y"=w319, "x"=w320) -> ("y out"=w322:dbl, "x out"=w321:dbl)  [unwired: 6 in, 1 out]
          n124 = Build Array(w321, w322, 0.0 ("element"), 0.0 ("element")) -> (w315:dbl[])
          n125 = Add(x=w315, y=w316) -> (x+y=w314:dbl[])
        }
      }
      event "Measure Pickup Tools": Value Change {
        (unwired) "Measuring Pickup Tools" ("String")
        n126 = event-data() -> ()  [unwired: 1 in, 6 out]
        n127 = for {
          N: w369 -> [_]
          tunnel: [w402] -> w377 mode=indexing
          tunnel: w378 -> [w406]
          tunnel: [w388] -> w376
          tunnel: w375 -> [w387] mode=indexing
          # "Default size and\norientation"
          n128 = call "Joystick and Camera - external Connection.vi"("Motion in"=w406, "XYZTheta"=w387, "Measurement Point"="PickUp tool Top") -> ("Motion out"=w382:refnum<class "Motion.lvclass">, "Sum"=w405:dbl[])  [unwired: 4 in, 2 out]
          n129 = Build Array(0.0 ("element"), 29.94 ("element"), 0.0 ("element"), 0.0 ("element")) -> (w393:dbl[])
          n130 = Add(x=w405, y=w393) -> (x+y=w379:dbl[])
          n131 = Array Subset(array=w379, index=0, length=2) -> (w380:dbl[])
          n132 = call-dynamic "XY Go.vi"("Speed"=20.0, "XY"=w380, "Motion in"=w382) -> ("Motion out"=w381:refnum<class "Motion.lvclass">)  [unwired: 7 in, 1 out]
          n133 = call "Joystick and Camera - external Connection.vi"("Motion in"=w381, "Measurement Point"="PickUp tool Bottom", "Inital GO"=FALSE) -> ("Motion out"=w388:refnum<class "Motion.lvclass">, "Sum"=w404:dbl[])  [unwired: 4 in, 2 out]
          n134 = Add(x=w405, y=w404) -> (x+y=w411:dbl[])
          n135 = Subtract(x=w404, y=w405) -> (x-y=w403:dbl[])
          n136 = Divide(x=w411, y=2.0) -> (x/y=w408:dbl[])
          n137 = call "XYtoRPHI.vi"("X-Y"=w403) -> ("r-phi"=w409:dbl[])
          n138 = Index Array(array=w409, index=1) -> (element=w397:dbl)
          n139 = Absolute Value(x=w397) -> (abs(x)=w400:dbl)
          n140 = Sign(1:w397) -> (0:w398:dbl)
          n141 = Subtract(x=w400, y=1.5707963267948966) -> (x-y=w399:dbl)
          n142 = Multiply(x=w398, y=w399) -> (x*y=w396:dbl)
          n143 = Replace Array Subset(array=w408, new element=w396, index=3) -> (w402:dbl[])
          "PickupTool \nCenterPosition" <- w402
        }
      }
      event "Deposit Glue": Value Change {
        # "CF height"
        # "surface z offset"
        # "two sensor, Sensor B then A"
        # "Unmount syringe"
        # "first needle park position\nneedle gap on Z value : 0.5 mm"
        # "Syringe-camera offset"
        n144 = event-data() -> ()  [unwired: 1 in, 6 out]
        n145 = call-poly <vilib>:"Read Delimited Spreadsheet.vi"("file path (dialog if empty)"=path "D:/INTT/V1/Assembly Data/Tool Offsets/Dispense Tip Offset.txt", "number of rows (all:-1)"=-1) -> ("first row"=w467:dbl[])  [unwired: 8 in, 5 out]
        n146 = Add(x=14.2 ("element"), y=w423) -> (x+y=w417:dbl)
        n147 = Index Array(array=w467, index #1=0 ("index"), index #2=1 ("index")) -> (element #1=w462:dbl, element #2=w460:dbl)
        n148 = Build Array(w462, w460, 0.0 ("element"), 0.0 ("element")) -> (w446:dbl[])
        n149 = Array Subset(array=w413, index (row)=0, length (row)=1 ("length")) -> (w426:dbl[][])  [unwired: 2 in]
        n150 = Reshape Array(w426, 4 ("dimension size")) -> (w419:dbl[])
        n151 = Index Array(array=w419, index=2) -> (element=w414:dbl)
        n152 = Add(x=w414, y=w417) -> (x+y=w416:dbl)
        n153 = Build Array(436.638, 1040.76, w416, 0.0 ("element")) -> (w415:dbl[])
        "Needle parking position" <- w415
        n154 = call "XYZTheta Go.vi"("XYZTheta In"=w415, "Motion in"=w451) -> ("error out"=w459:errorcluster, "Motion out"=w450:refnum<class "Motion.lvclass">)  [unwired: 7 in, 1 out]
        n155 = call "Display Message to User"("error in (no error)"=w459) -> ("error out"=w452:errorcluster)  [unwired: 9 in, 1 out]
        n156 = call-dynamic "Z Go.vi"("error in (no error)"=w452, "Speed"=20.0, "Position"=0.0, "Motion in"=w450) -> ("error out"=w449:errorcluster, "Motion out"=w455:refnum<class "Motion.lvclass">)  [unwired: 6 in]
        n157 = case shown="False" w421 {
          tunnel: w413 -> [w475 w484]
          tunnel: [w472 w484] -> w420
          frame False {
            n158 = Array Subset(array=w475, index (row)=1 ("index"), length (row)=1 ("length")) -> (w476:dbl[][])  [unwired: 2 in]
            n159 = Array Subset(array=w475, index (row)=0 ("index"), length (row)=1 ("length")) -> (w479:dbl[][])  [unwired: 2 in]
            n160 = Reshape Array(w479, 4 ("dimension size")) -> (w474:dbl[])
            n161 = Reshape Array(w476, 4 ("dimension size")) -> (w473:dbl[])
            n162 = Build Array(w473, w474) -> (w472:dbl[][])
          }
          frame True {
          }
        }
        n163 = call "Display Message to User2"("error in (no error)"=w449) -> ("error out"=w448:errorcluster)  [unwired: 9 in, 1 out]
        n164 = Add(x=w414, y=-2.5) -> (x+y=w456:dbl)
        n165 = call-dynamic "Z Go.vi"("error in (no error)"=w448, "Speed"=20.0, "Position"=w456, "Motion in"=w455) -> ("error out"=w425:errorcluster, "Motion out"=w447:refnum<class "Motion.lvclass">)  [unwired: 6 in]
        n166 = call-dynamic "Connect.vi"("Ultimus V in"=refnum<class "Ultimus V2.lvclass"> refnum ("Ultimus V2.lvclass")) -> ("Ultimus V out"=w445:refnum<class "Ultimus V2.lvclass">)  [unwired: 9 in, 1 out]
        n167 = for {
          N: w440 -> [_]
          tunnel: w447 -> [w499]
          tunnel: w445 -> [w498]
          tunnel: w446 -> [w500]
          tunnel: w435 -> [_] mode=indexing
          tunnel: w420 -> [w501] mode=indexing
          tunnel: [w497] -> w433
          tunnel: [w496] -> w432
          tunnel: w425 -> [w492]
          tunnel: [w493] -> w424
          tunnel: w422 -> [w491]
          (unwired) 100.0 ("Speed")
          n168 = Add(x=w501, y=w500) -> (x+y=w531:dbl[])
          n169 = Add(x=w531, y=dbl[] [3.3, 5.0, 0.0, 0.0]) -> (x+y=w532:dbl[])
          n170 = Index Array(array=w532, index=2) -> (element=w489:dbl)
          n171 = Array Subset(array=w532, index=0, length=2) -> (w507:dbl[])
          n172 = call-dynamic "XY Go.vi"("error in (no error)"=w492, "Speed"=100.0, "XY"=w507, "Motion in"=w499) -> ("error out"=w487:errorcluster, "Motion out"=w488:refnum<class "Motion.lvclass">)  [unwired: 6 in]
          n173 = case shown="True" "check height?" {
            tunnel: w489 -> [_ w548]
            tunnel: w488 -> [w541 w547]
            tunnel: w487 -> [w542 w546]
            tunnel: [w542 w544] -> w486
            tunnel: [w541 w543] -> w485
            frame False {
            }
            frame True {
              n174 = call-dynamic "Z Go.vi"("error in (no error)"=w546, "Speed"=5.0, "Position"=w548, "Motion in"=w547) -> ("error out"=w545:errorcluster, "Motion out"=w543:refnum<class "Motion.lvclass">)  [unwired: 6 in]
              n175 = call "Display Message to User4"("error in (no error)"=w545) -> ("error out"=w544:errorcluster)  [unwired: 9 in, 1 out]
            }
          }
          n176 = Add(x=w489, y=-2.0) -> (x+y=w506:dbl)
          n177 = call-dynamic "Z Go.vi"("error in (no error)"=w486, "Speed"=5.0, "Position"=w506, "Motion in"=w485) -> ("error out"=w504:errorcluster, "Motion out"=w505:refnum<class "Motion.lvclass">)  [unwired: 6 in]
          n178 = call "Muliti_XY_dispense.vi"("Pressure"=w491, "Path count"=4, "distances"=dbl[][] [[0.0, 224.0], [27.4, 0.0], [0.0, -224.0], [-27.4, 0.0]], "Ultimus V in"=w498, "Motion in"=w505) -> ("Ultimus V out"=w525:refnum<class "Ultimus V2.lvclass">, "Motion out"=w530:refnum<class "Motion.lvclass">)  [unwired: 5 in]
          n179 = call-dynamic "wrtCurrent Go.vi"("axis names"=string[] ["X", "Y"], "error in (no error)"=w504, "Speed"=5.0, "distances"=dbl[] [4.6, 5.0], "Motion in"=w530) -> ("error out"=w495:errorcluster, "Motion out"=w524:refnum<class "Motion.lvclass">)  [unwired: 5 in]
          n180 = call "Muliti_XY_dispense.vi"("Pressure"=w491, "Path count"=4, "distances"=dbl[][] [[0.0, 214.0], [18.2, 0.0], [0.0, -214.0], [-18.2, 0.0]], "Ultimus V in"=w525, "Motion in"=w524) -> ("Ultimus V out"=w517:refnum<class "Ultimus V2.lvclass">, "Motion out"=w516:refnum<class "Motion.lvclass">)  [unwired: 5 in]
          n181 = call-dynamic "wrtCurrent Go.vi"("axis names"=string[] ["X", "Y"], "error in (no error)"=w495, "Speed"=5.0, "distances"=dbl[] [4.6, 5.0], "Motion in"=w516) -> ("error out"=w494:errorcluster, "Motion out"=w515:refnum<class "Motion.lvclass">)  [unwired: 5 in]
          n182 = call "Muliti_XY_dispense.vi"("Pressure"=w491, "Path count"=4, "distances"=dbl[][] [[0.0, 204.0], [9.0, 0.0], [0.0, -204.0], [-9.0, 0.0]], "Ultimus V in"=w517, "Motion in"=w515) -> ("Ultimus V out"=w502:refnum<class "Ultimus V2.lvclass">, "Motion out"=w503:refnum<class "Motion.lvclass">)  [unwired: 5 in]
          n183 = call-dynamic "wrtCurrent Go.vi"("axis names"=string[] ["X", "Y"], "error in (no error)"=w494, "Speed"=5.0, "distances"=dbl[] [4.5, 5.0], "Motion in"=w503) -> ("error out"=w493:errorcluster, "Motion out"=w509:refnum<class "Motion.lvclass">)  [unwired: 5 in]
          n184 = call "Muliti_XY_dispense.vi"("Pressure"=w491, "Path count"=1, "distances"=dbl[][] [[0.0, 194.0], [7.0, 0.0], [0.0, -206.0], [-7.0, 0.0]], "Ultimus V in"=w502, "Motion in"=w509) -> ("Ultimus V out"=w496:refnum<class "Ultimus V2.lvclass">, "Motion out"=w497:refnum<class "Motion.lvclass">)  [unwired: 5 in]
        }
        n185 = call "XYZTheta Go.vi"("error in (no error)"=w424, "XYZTheta In"=dbl[] [500.0, 1000.0, 0.0, 0.1], "Motion in"=w433) -> ("error out"=w443:errorcluster, "Motion out"=w441:refnum<class "Motion.lvclass">)  [unwired: 6 in, 1 out]
        n186 = call "Display Message to User3"("error in (no error)"=w443) -> ()  [unwired: 9 in, 2 out]
        n187 = call-dynamic "Disconnect.vi"("Ultimus V in"=w432) -> ()  [unwired: 9 in, 1 out]
      }
      event "Needle Alignment": Value Change {
        (unwired) "Needle Alignment in progress ...." ("String")
        # "CF height"
        # "surface z offset"
        # "first needle park position\nneedle gap on Z value : 0.5 mm"
        # "Syringe-camera offset"
        n188 = event-data() -> ()  [unwired: 1 in, 6 out]
        n189 = Array Subset(array=w551, index (row)=0, length (row)=1 ("length")) -> (w554:dbl[][])  [unwired: 2 in]
        n190 = Reshape Array(w554, 4 ("dimension size")) -> (w553:dbl[])
        n191 = Index Array(array=w553, index=2) -> (element=w550:dbl)
        n192 = call-poly <vilib>:"Read Delimited Spreadsheet.vi"("file path (dialog if empty)"=path "D:/INTT/V1/Assembly Data/Tool Offsets/Dispense Tip Offset.txt", "number of rows (all:-1)"=-1) -> ("first row"=w601:dbl[])  [unwired: 8 in, 5 out]
        n193 = Index Array(array=w601, index #1=0 ("index"), index #2=1 ("index")) -> (element #1=w596:dbl, element #2=w595:dbl)
        n194 = Add(x=14.2 ("element"), y=w559) -> (x+y=w561:dbl)
        n195 = Add(x=w550, y=w561) -> (x+y=w560:dbl)
        n196 = Build Array(436.638, 1040.76, w560, 0.0 ("element")) -> (w558:dbl[])
        n197 = Build Array(w596, w595, 0.0 ("element"), 0.0 ("element")) -> (w570:dbl[])
        n198 = call "XYZTheta Go.vi"("XYZTheta In"=w558, "Motion in"=w585) -> ("error out"=w594:errorcluster, "XYZTheta Out"=w575:dbl[], "Motion out"=w584:refnum<class "Motion.lvclass">)  [unwired: 7 in]
        n199 = call "Display Message to User10"("error in (no error)"=w594) -> ("error out"=w591:errorcluster)  [unwired: 9 in, 1 out]
        n200 = call-dynamic "Z Go.vi"("error in (no error)"=w591, "Speed"=20.0, "Position"=0.0, "Motion in"=w584) -> ("Motion out"=w583:refnum<class "Motion.lvclass">)  [unwired: 6 in, 1 out]
        n201 = Replace Array Subset(array=w575, new element=0.0 ("new element/subarray"), index=2) -> (w572:dbl[])
        n202 = call "Joystick and Camera - external Connection.vi"("Motion in"=w583, "XYZTheta"=w572, "Measurement Point"="Touch Needle on a surface") -> ("Motion out"=w581:refnum<class "Motion.lvclass">, "Gantry"=w571:dbl[])  [unwired: 4 in, 2 out]
        n203 = Subtract(x=w571, y=w570) -> (x-y=w569:dbl[])
        n204 = call "Joystick and Camera - external Connection.vi"("Motion in"=w581, "XYZTheta"=w569, "Measurement Point"="Measure the touch spot with camera") -> ("Motion out"=w577:refnum<class "Motion.lvclass">, "Gantry"=w580:dbl[])  [unwired: 4 in, 2 out]
        n205 = Subtract(x=w571, y=w580) -> (x-y=w579:dbl[])
        n206 = call-poly <vilib>:"Write Delimited Spreadsheet.vi"("file path (dialog if empty)"=path "D:/INTT/V1/Assembly Data/Tool Offsets/Dispense Tip Offset.txt", "1D data"=w579, "append to file? (new file:F)"=FALSE) -> ()  [unwired: 11 in, 2 out]
      }
      event "Pick and place": Value Change {
        (unwired) "PICK and PLACE samples ..." ("String")
        n207 = event-data() -> ()  [unwired: 1 in, 6 out]
        n208 = case shown="False" w605 {
          tunnel: w609 -> [w631 w653]
          tunnel: [w630 w652] -> w608
          frame False {
            n209 = Array Subset(array=w631, index (row)=0 ("index"), length (row)=1 ("length")) -> (w633:dbl[][])  [unwired: 2 in]
            n210 = Build Array(11.75 ("element"), 173.55 ("element"), 0.0 ("element"), 0.0 ("element")) -> (w637:dbl[])
            n211 = Reshape Array(w633, 4 ("dimension size")) -> (w632:dbl[])
            n212 = Add(x=w637, y=w632) -> (x+y=w630:dbl[])
          }
          frame True {
            n213 = Array Subset(array=w653, index (row)=0 ("index"), length (row)=1 ("length")) -> (w643:dbl[][])  [unwired: 2 in]
            n214 = Build Array(11.75 ("element"), 56.85 ("element"), 0.0 ("element"), 0.0 ("element")) -> (w647:dbl[])
            n215 = Reshape Array(w643, 4 ("dimension size")) -> (w642:dbl[])
            n216 = Add(x=w647, y=w642) -> (x+y=w652:dbl[])
          }
        }
        n217 = call-poly <vilib>:"Read Delimited Spreadsheet.vi"("file path (dialog if empty)"=path "D:/INTT/V1/Assembly Data/Tool Offsets/Bellows Tool Offset.txt", "number of rows (all:-1)"=-1) -> ("first row"=w626:dbl[])  [unwired: 8 in, 5 out]
        n218 = Index Array(array=w626, index #1=0 ("index"), index #2=1 ("index"), index #3=2 ("index")) -> (element #1=w622:dbl, element #2=w621:dbl, element #3=w620:dbl)
        n219 = for {
          N: 1 -> [_]
          tunnel: w629 -> [w659]
          tunnel: [w681] -> w619
          tunnel: w618 -> [w690] mode=indexing
          tunnel: [w668] -> w612
          tunnel: w613 -> [w658]
          tunnel: w622 -> [w683]
          tunnel: w621 -> [w682]
          tunnel: w620 -> [w680]
          tunnel: w614 -> [w674]
          tunnel: w611 -> [w661]
          tunnel: w608 -> [w660]
          tunnel: w606 -> [w656]
          w670 = 0 ("Write")
          w673 = TRUE ("Write Value")
          # "putback pickup tool"
          # "pickup tool"
          # "pickup tool height offset"
          # "Pick up PICKUP TOOL"
          # "Pick up CHIPs/Sensor and place on HDI"
          n220 = Build Array(w683, w682, w680, 0.0 ("element")) -> (w679:dbl[])
          n221 = Add(x=w690, y=w679) -> (x+y=w654:dbl[])
          n222 = call "XYZTheta-2Zspeed Go.vi"("XYZTheta In"=w654, "Motion in"=w659) -> ("error out"=w657:errorcluster, "Motion out"=w655:refnum<class "Motion.lvclass">)  [unwired: 7 in, 1 out]
          n223 = Replace Array Subset(array=w679, new element=-16.0 ("t"), index=2) -> (w677:dbl[])
          n224 = call "WriteReadWait.vi"("Read Value"=w673, "Write Value"=w673, "error in (no error)"=w657, "Read"=w670, "Write"=w670, "I-O in"=w658) -> ("error out"=w672:errorcluster, "I-O out"=w671:refnum<class "NI-DAQ.lvclass">)  [unwired: 4 in]
          n225 = for {
            N: w674 -> [_]
            tunnel: w655 -> [w702]
            tunnel: w677 -> [w701]
            tunnel: w672 -> [w700]
            tunnel: [w699] -> w684
            tunnel: w671 -> [w698]
            tunnel: [w697] -> w669
            tunnel: [w696] -> w676
            tunnel: w661 -> [w693]
            tunnel: w660 -> [w692]
            tunnel: w656 -> [w691] mode=indexing
            n226 = flat-sequence {
              tunnel: [w721] -> w703
              tunnel: w702 -> [w720]
              tunnel: w701 -> [w719]
              tunnel: w700 -> [w717]
              tunnel: w698 -> [w709]
              tunnel: [w716] -> w695
              tunnel: [w713] -> w694
              tunnel: w693 -> [w706]
              tunnel: w692 -> [w712]
              tunnel: w703 -> [w725]
              tunnel: [w735] -> w699
              tunnel: [w734] -> _
              tunnel: w701 -> [w727]
              tunnel: [w728] -> w697
              tunnel: [w723] -> w696
              tunnel: w695 -> [w730]
              tunnel: w694 -> [w724]
              tunnel: w691 -> [w726]
              frame #0 {
                w707 = FALSE ("Write Value")
                w714 = TRUE ("Write Value")
                w715 = 1 ("Write")
                # "pickup module"
                # "release module"
                # "pickup sample from tray"
                n227 = Add(x=w712, y=w719) -> (x+y=w718:dbl[])
                n228 = call "XYZTheta-2Zspeed Go.vi"("error in (no error)"=w717, "XYZTheta In"=w718, "Motion in"=w720) -> ("error out"=w710:errorcluster, "Motion out"=w721:refnum<class "Motion.lvclass">)  [unwired: 6 in, 1 out]
                n229 = call "Time Delay"("error in (no error)"=w710) -> ("error out"=w705:errorcluster)  [unwired: 10 in]
                n230 = call "WriteReadWait.vi"("Read Value"=w707, "Write Value"=w707, "error in (no error)"=w705, "Read"=w706, "Write"=w706, "I-O in"=w709) -> ("error out"=w704:errorcluster, "I-O out"=w708:refnum<class "NI-DAQ.lvclass">)  [unwired: 4 in]
                n231 = call "Time Delay3"("error in (no error)"=w704) -> ("error out"=w711:errorcluster)  [unwired: 10 in]
                n232 = call "WriteReadWait.vi"("Read Value"=w714, "Write Value"=w714, "error in (no error)"=w711, "Read"=w715, "Write"=w715, "I-O in"=w708) -> ("error out"=w713:errorcluster, "I-O out"=w716:refnum<class "NI-DAQ.lvclass">)  [unwired: 4 in]
              }
              frame #1 {
                w729 = 1 ("Write")
                w731 = FALSE ("Write Value")
                # "lift for chip/sensor thickness"
                # "place sample on HDI"
                n233 = Add(x=w726, y=w727) -> (x+y=w722:dbl[])
                n234 = call "XYZTheta-2Zspeed Go.vi"("error in (no error)"=w724, "XYZTheta In"=w722, "Motion in"=w725) -> ("error out"=w733:errorcluster, "XYZTheta Out"=w734:dbl[], "Motion out"=w735:refnum<class "Motion.lvclass">)  [unwired: 6 in]
                n235 = call "Time Delay6"("error in (no error)"=w733) -> ("error out"=w732:errorcluster)  [unwired: 10 in]
                n236 = call "WriteReadWait.vi"("Read Value"=w731, "Write Value"=w731, "error in (no error)"=w732, "Read"=w729, "Write"=w729, "I-O in"=w730) -> ("error out"=w723:errorcluster, "I-O out"=w728:refnum<class "NI-DAQ.lvclass">)  [unwired: 4 in]
              }
            }
          }
          n237 = call "XYZTheta-2Zspeed Go.vi"("error in (no error)"=w676, "XYZTheta In"=w654, "Motion in"=w684) -> ("error out"=w664:errorcluster, "Motion out"=w688:refnum<class "Motion.lvclass">)  [unwired: 6 in, 1 out]
          n238 = call "Time Delay9"("error in (no error)"=w664) -> ("error out"=w666:errorcluster)  [unwired: 10 in]
          n239 = call-dynamic "Digital Write 1 Channel.vi"("DAQ Module"=0, "error constant"=w666, "Value"=FALSE, "Channel"=0, "NI-DAQ.lvclass"=w669) -> ("error IO"=w665:errorcluster, "NI-DAQ.lvclass 2"=w668:refnum<class "NI-DAQ.lvclass">)  [unwired: 5 in]
          n240 = call "Time Delay10"("error in (no error)"=w665) -> ("error out"=w685:errorcluster)  [unwired: 10 in]
          n241 = call-dynamic "Z Go.vi"("error in (no error)"=w685, "Speed"=10.0, "Position"=0.0 ("new element/subarray"), "Motion in"=w688) -> ("Motion out"=w681:refnum<class "Motion.lvclass">)  [unwired: 6 in, 1 out]
        }
      }
      event "GOTO": Value Change {
        (unwired) "GOING to a position" ("String")
        n242 = event-data() -> ()  [unwired: 1 in, 6 out]
        n243 = call "XYZTheta Go.vi"("XYZTheta In"="Parking position", "Motion in"=w741) -> ("Motion out"=w739:refnum<class "Motion.lvclass">)  [unwired: 7 in, 2 out]
      }
      event "READ Position": Value Change {
        n244 = event-data() -> ()  [unwired: 1 in, 6 out]
        n245 = call-dynamic "Get Current Position.vi"("Motion in"=w759) -> ("XYZTheta Out"=→"Gantry current position":dbl[], "Motion out"=w758:refnum<class "Motion.lvclass">)  [unwired: 8 in, 1 out]
      }
      event "HDI vacuum": Value Change {
        n246 = event-data() -> ()  [unwired: 1 in, 6 out]
        n247 = call "WriteReadWait.vi"("Read Value"="vacuum", "Write Value"="vacuum", "Read"=w770, "Write"=w770, "I-O in"=w773) -> ("error out"=w771:errorcluster, "I-O out"=w760:refnum<class "NI-DAQ.lvclass">)  [unwired: 5 in]
        n248 = call "Time Delay2"("error in (no error)"=w771) -> ()  [unwired: 10 in, 1 out]
      }
      event Timeout {
        n249 = event-data() -> ()  [unwired: 1 in, 3 out]
        n250 = call-dynamic "Digital Read 1 Channel.vi"("Read"=w784, "NI-DAQ in"=w785) -> ("Value"=→"Status":bool, "NI-DAQ out"=w783:refnum<class "NI-DAQ.lvclass">)  [unwired: 7 in, 1 out]
      }
    }
    "Measured HDI size" <- w17
    "module position on stave" <- w18
    "Stave mark" <- w16
    "measured HDI top-left position" <- w13
    n251 = feedback-in #1(w17) -> ()
    n252 = feedback-in #2(w16) -> ()
    n253 = feedback-in #3(w13) -> ()
    n254 = feedback-in #4(w29) -> ()
    n255 = feedback-in #5(w26) -> ()
    n256 = feedback-in #6(w34) -> ()
    n257 = feedback-in #7(w18) -> ()
    n258 = feedback-in #8(w35) -> ()
    "# of tasks excuted" <- w31
  }
  n259 = call-dynamic "Disconnect.vi"("Controller in"=w4) -> ()  [unwired: 9 in, 1 out]
  n260 = call-dynamic "Disconnect.vi"("I-O in"=w1) -> ()  [unwired: 9 in, 1 out]
